vi "滑移力复检.vi"() -> ()   [LabVIEW 2020]
uses:
  <vilib>/Utility/miscctls.llb/LVRowAndColumnTypeDef.ctl
  Global_Variable/Global.vi
  Database/Global1.vi
  <vilib>/addons/database/Connection.llb/DB Tools Open Connec (String).vi
  Global_Variable/A131258.vi
  <vilib>/addons/database/Connection.llb/Conn Execute.vi
  <vilib>/addons/database/Recordset.llb/Rec Fetch Recordset Data (R).vi
  <vilib>/Utility/config.llb/NI_LVConfig.lvlib
  <vilib>/addons/database/NI_Database_API.lvlib
panel:
  out "判定":string[][](table)
  in  "滑移力判定项 2":string[][](table)
  out "连接的字符串 2":string
  out "连接的字符串":string
  out "时间":string
  out "前序工位":string[](array[string])
  out "二维码":string[][](array[string])
  out "传感器码":string[][](array[string])
  out "数组":refnum<vi>[](array[refnum])
  out "Fproductid_MAIN":string
  out "Fproductid_SENSOR":string
  out "USER_ID":string
  out "deviceid":string
  out "productid":string
  out "产品型号":string
  out "CODE_ID 2":string
  out "CODE_ID":string
  out "联机模式":string
  out "用户权限":string
  out "用户名":string
  in  "管柱合成报表":string[][](table)=[["mm"], ["mm/s"]]
  in  "拉轴判定结果":bool[][](array[boolean])=[[TRUE]]
  in  "滑移力判定结果":bool[][](array[boolean])=[[TRUE]]
  in  "管柱合成报表":string[][](table)=[["mm"], ["mm/s"]]
  in  "选项卡控件 2":enum32{"管柱总成装配", "管柱总成装配右", "滑移力曲线", "参数查看"}(tab)
  out "上柱管上序状态":string
  out "传感器上序状态":string
  out "上柱管上序状态":bool
  out "传感器上序状态":bool
  in  "质量报警":bool
  in  "设备缺料":bool
  in  "设备故障":bool
  out "产品条码":string
  out "不合格指示灯":bool
  out "合格指示灯":bool
  out "产品条码 3":string
  out "上柱管上序状态 3":string
  out "传感器上序状态 3":string
  out "上柱管上序状态 2":bool
  out "传感器上序状态 2":bool
  in  "质量报警2":bool
  in  "设备缺料2":bool
  in  "设备故障2":bool
  out "产品条码 2":string
  out "不合格指示灯":bool
  out "合格指示灯":bool
  out "产品条码 4":string
  out "装配结果":string
  out "管柱码状态":string
  out "传感器码状态":string
  out "管柱二维码":string
  out "传感器码":string
  out "滑移力复检曲线":cluster{dbl[], dbl[]}[](graph)
  out "表格控件":string[][](table)
  in  "删除":bool
  in  "确定":bool
  in  "添加":bool
  in  "退出":bool
  in  "更新":bool
  in  "产品型号":string(combo)
  in  "选项卡控件 3":enum32{"产品管理", "用户管理", "判定参数"}(tab)
  in  "请输入添加的产品名称":string
  in  "请选择要删除的产品":string(combo)
  in  "进入用户管理":bool
  in  "坐标参数":string[][](table)
  in  "滑移力判定项":string[][](table)
  in  "压力判定项":string[][](table)
  in  "判定项":string[][](table)=[["MM", "130", "180", ""], ["N", "-60", "-10", ""], ["N", "-60", "-10", ""], ["", "", "", ""], ["", "", "", ""], ["", "", "", ""]]
  # "滑移力复测及管柱总成装配台"
  # "产品二维码"
  # "生产结果"
  # "看板呼叫"
  # "壳体二维码"
  # "上序状态："
  # "上柱管二维码"
  # "上序状态："
  # "产品二维码"
  # "生产结果"
  # "看板呼叫"
  # "壳体二维码"
  # "上序状态："
  # "上柱管二维码"
  # "上序状态："
  # "装配结果"
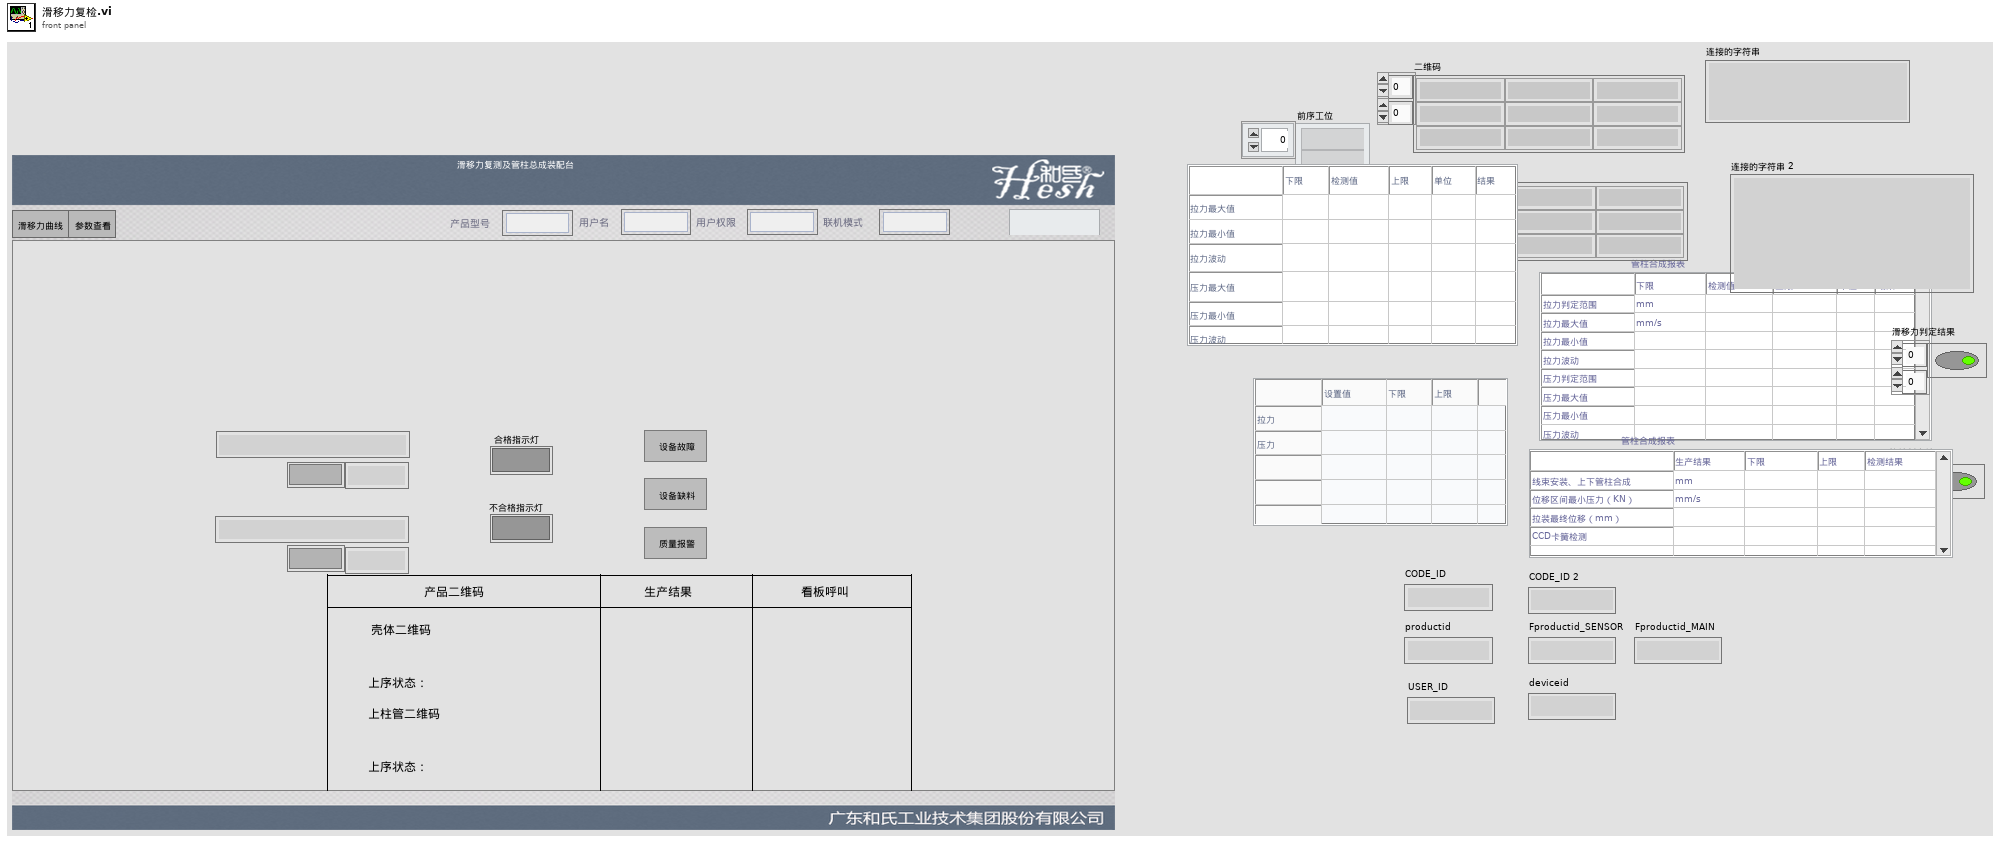
[diagram p1: front panel]
types:
  T1 = typedef "LVRowAndColumnTypeDef.ctl" = cluster{"Row":i32, "Column":i32}
  T2 = enum32{"Invalid", "Standard", "Closed", "Hidden", "Minimized", "Maximized"}
  T3 = cluster{"用户编号":string, "用户名":string, "用户密码(密文)":string, "用户权限":string}
  T4 = cluster{"设备名称":string, "用户名":string, "设备状态":enum16{"设备离线", "设备正常", "设备缺料", "设备故障", "质量报警"}, "附加信息":string}
  T5 = typedef "NI_LVConfig.lvlib/Config Data RefNum.ctl" = refnum<k1>
  T6 = typedef "NI_Database_API.lvlib/Conn ObjectReference.ctl" = refnum<k1>
  T7 = cluster{i64, i64, string, dbl, dbl, dbl, string, string}
  T8 = cluster{i64, i64, i64, string, "result string":string}
  T9 = cluster{i64, i64, i64, string, "result string":string}[]
  T10 = cluster{"拉力判定范围":cluster{"单位":string, "下限":dbl, "上限":dbl}, "拉力最大值":cluster{"单位":string, "下限":dbl, "上限":dbl}, "拉力最小值":cluster{"单位":string, "下限":dbl, "上限":dbl}, "拉力波动":cluster{"单位":string, "下限":dbl, "上限":dbl}, "压力判定范围":cluster{"单位":string, "下限":dbl, "上限":dbl}, "压力最大值":cluster{"单位":string, "下限":dbl, "上限":dbl}, "压力最小值":cluster{"单位":string, "下限":dbl, "上限":dbl}, "压力波动":cluster{"单位":string, "下限":dbl, "上限":dbl}}
  T11 = cluster{i64, i64, string, dbl, dbl, dbl, string, string}[]
  T12 = typedef "NI_Database_API.lvlib/Rec ObjectReference.ctl" = refnum<k1>
  T13 = cluster{"[0]":cluster{string, dbl, dbl}, "[1]":cluster{string, dbl, dbl}, "[2]":cluster{string, dbl, dbl}, "[3]":cluster{string, dbl, dbl}, "[4]":cluster{string, dbl, dbl}, "[5]":cluster{string, dbl, dbl}, "[6]":cluster{string, dbl, dbl}, "[7]":cluster{string, dbl, dbl}}
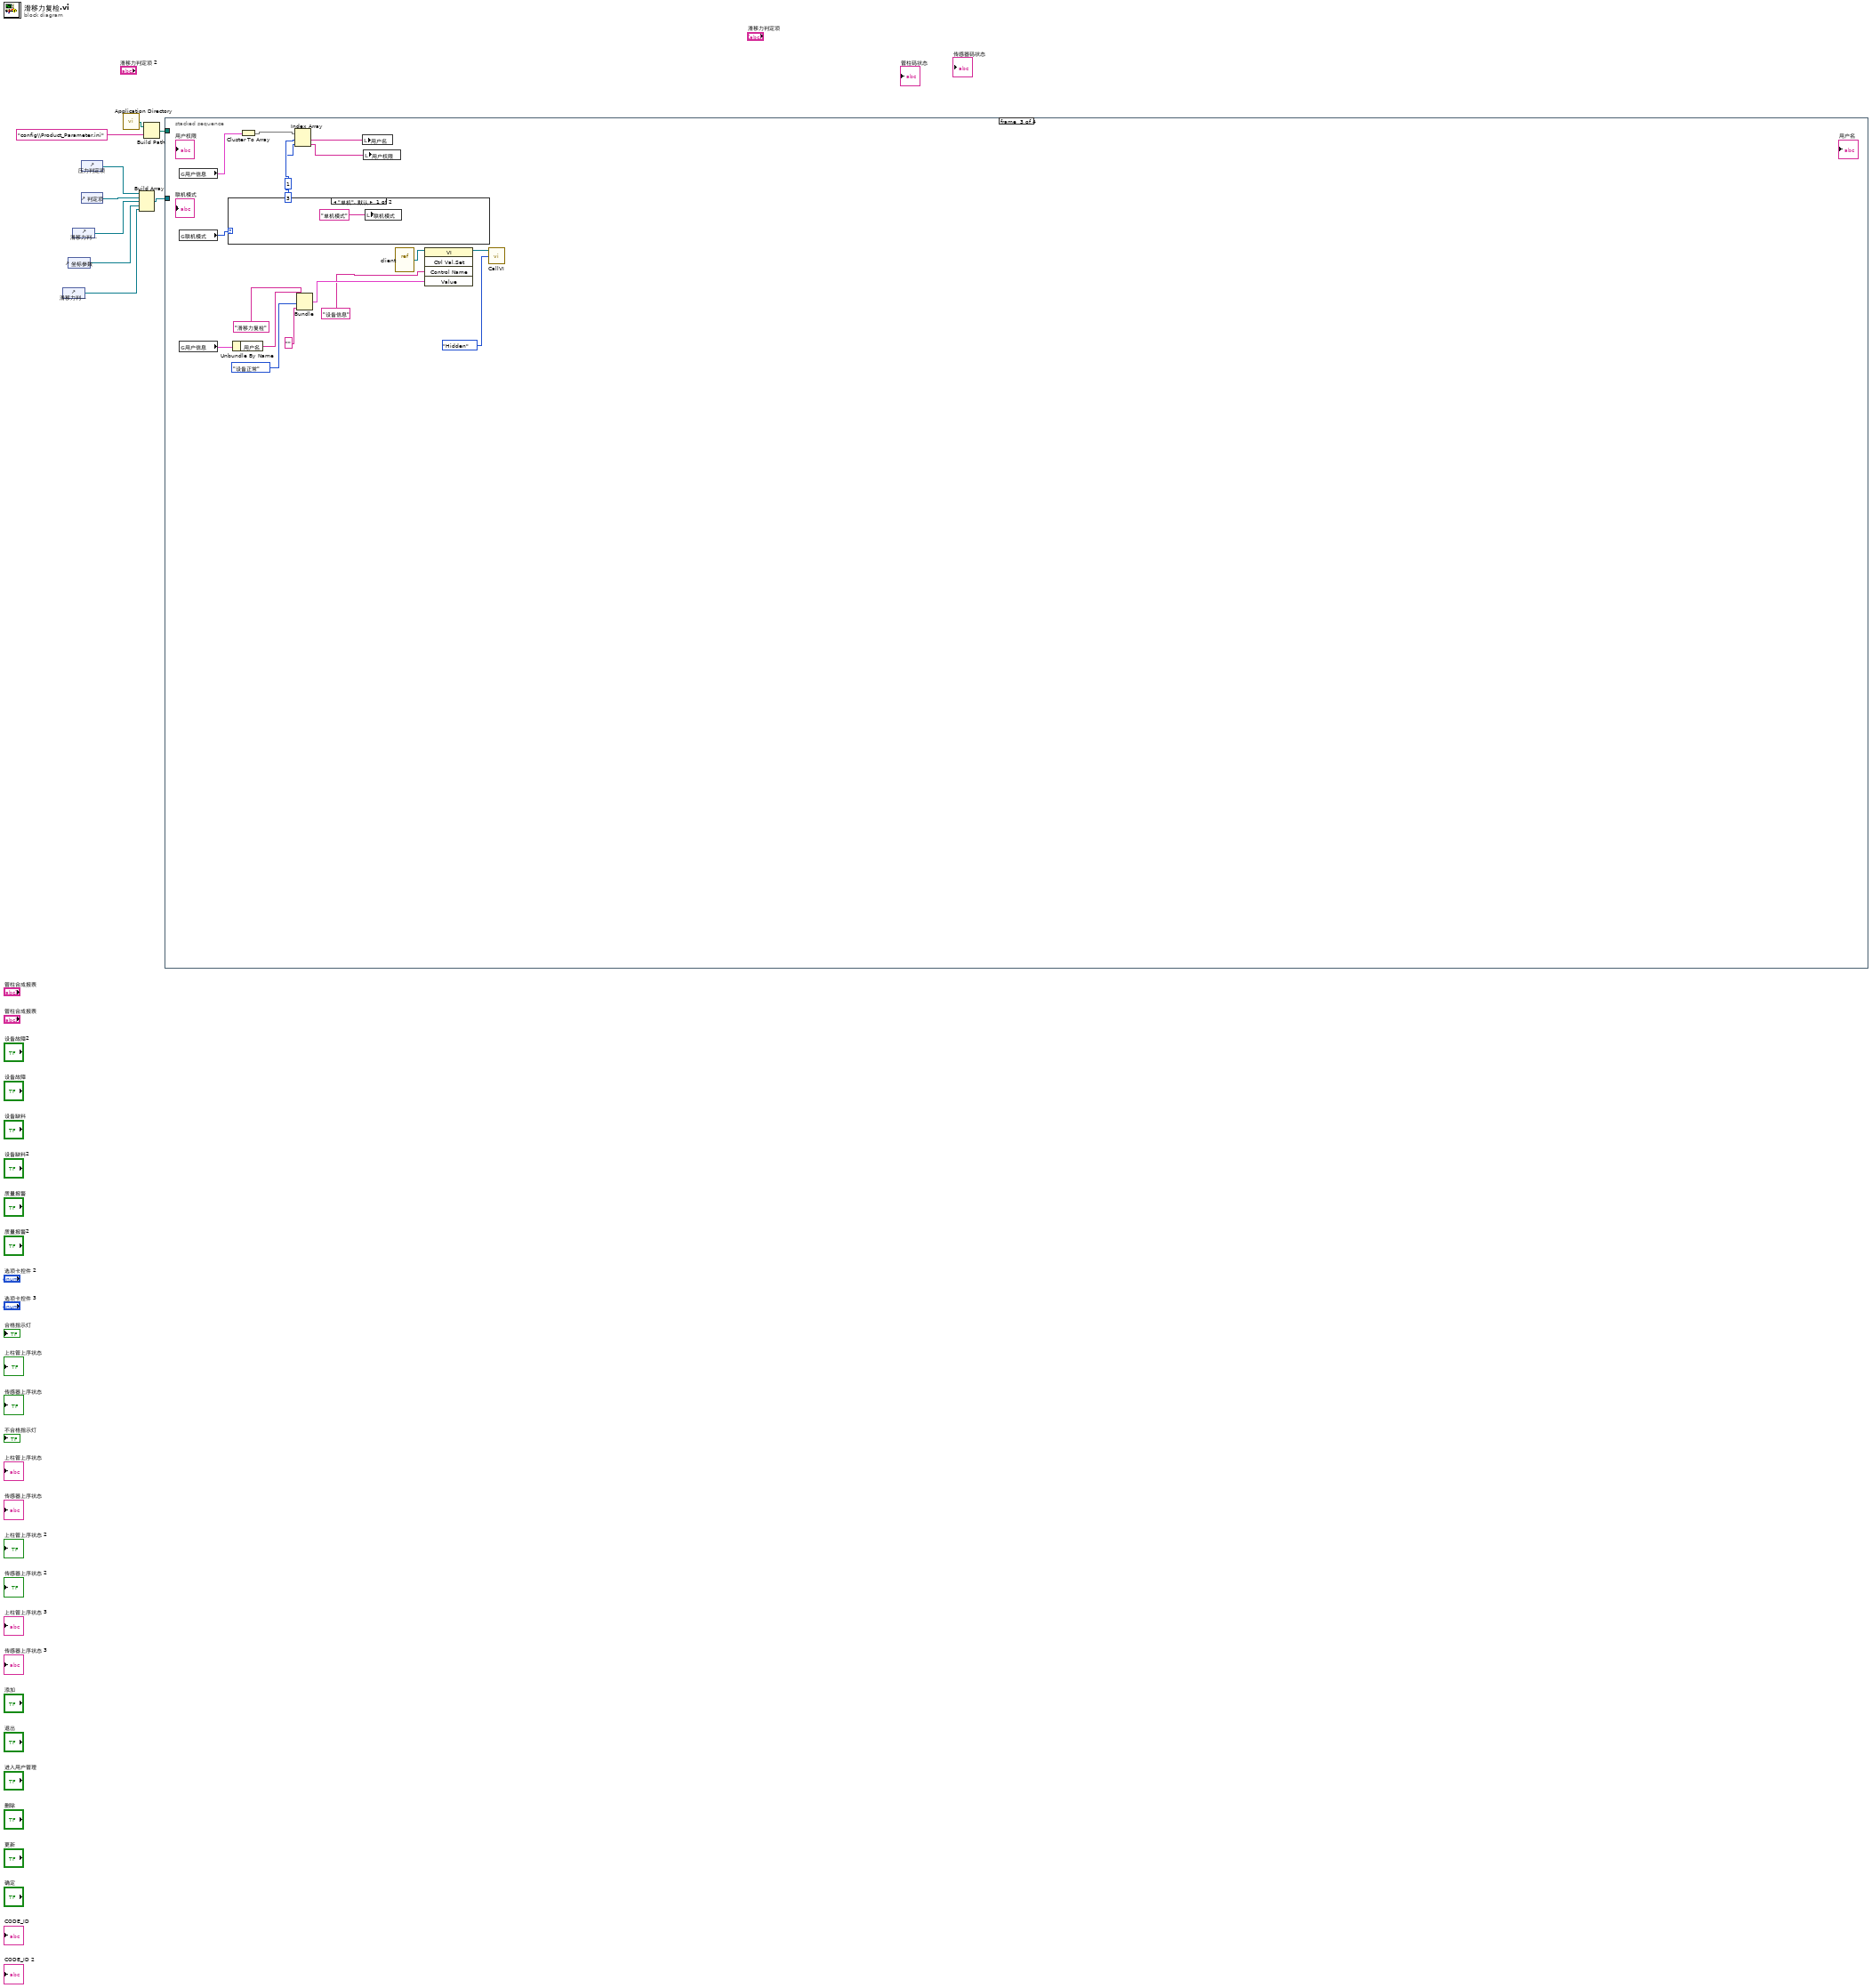
[diagram p0: block diagram]
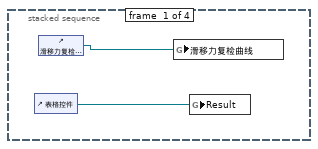
[diagram p2: hidden frame]
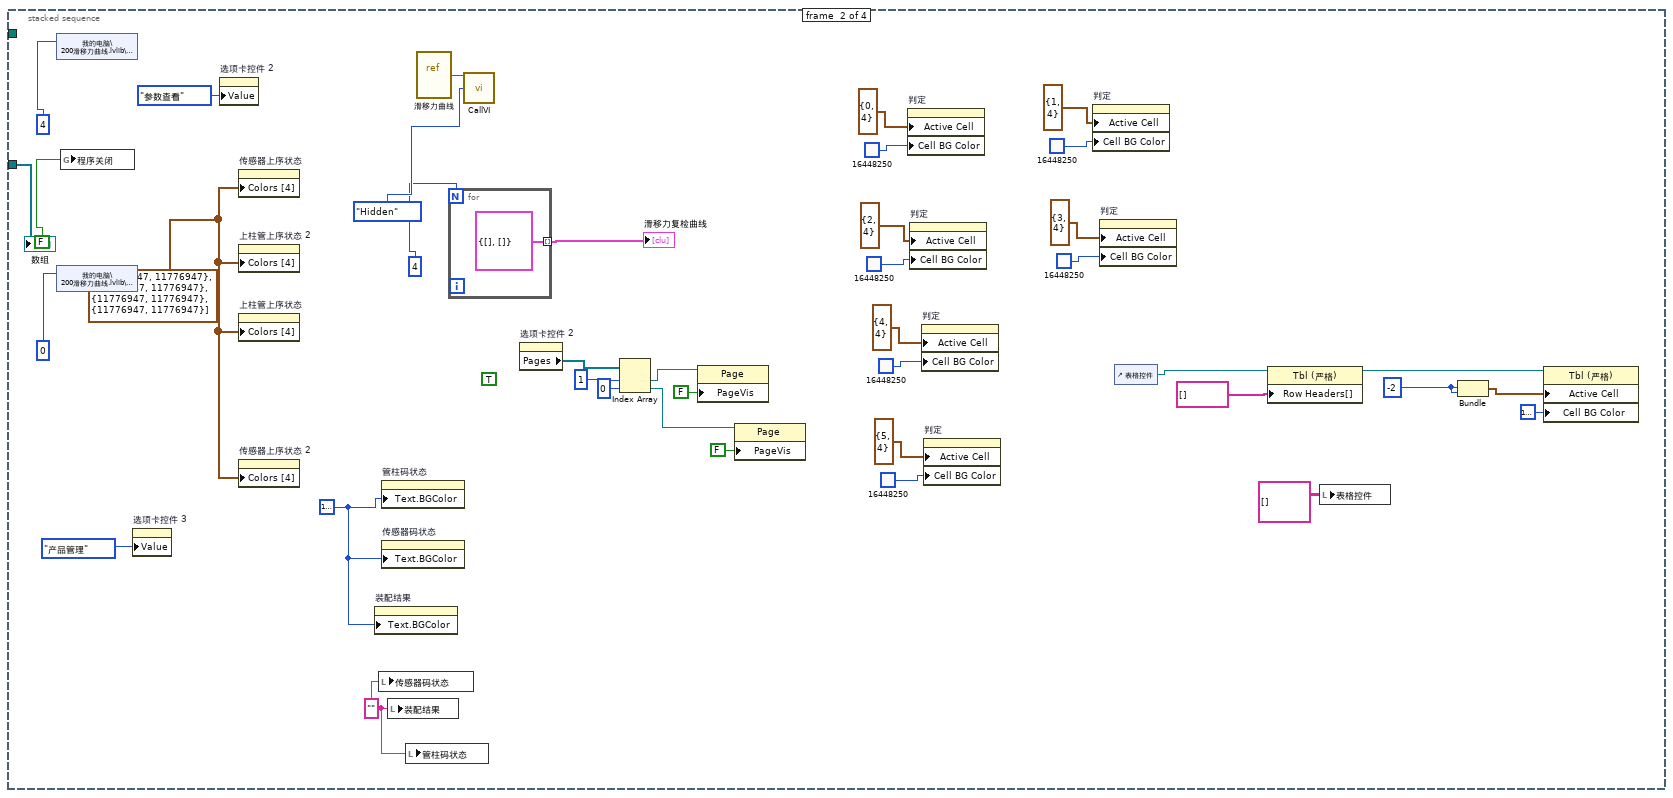
[diagram p3: hidden frame]
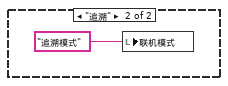
[diagram p4: hidden frame]
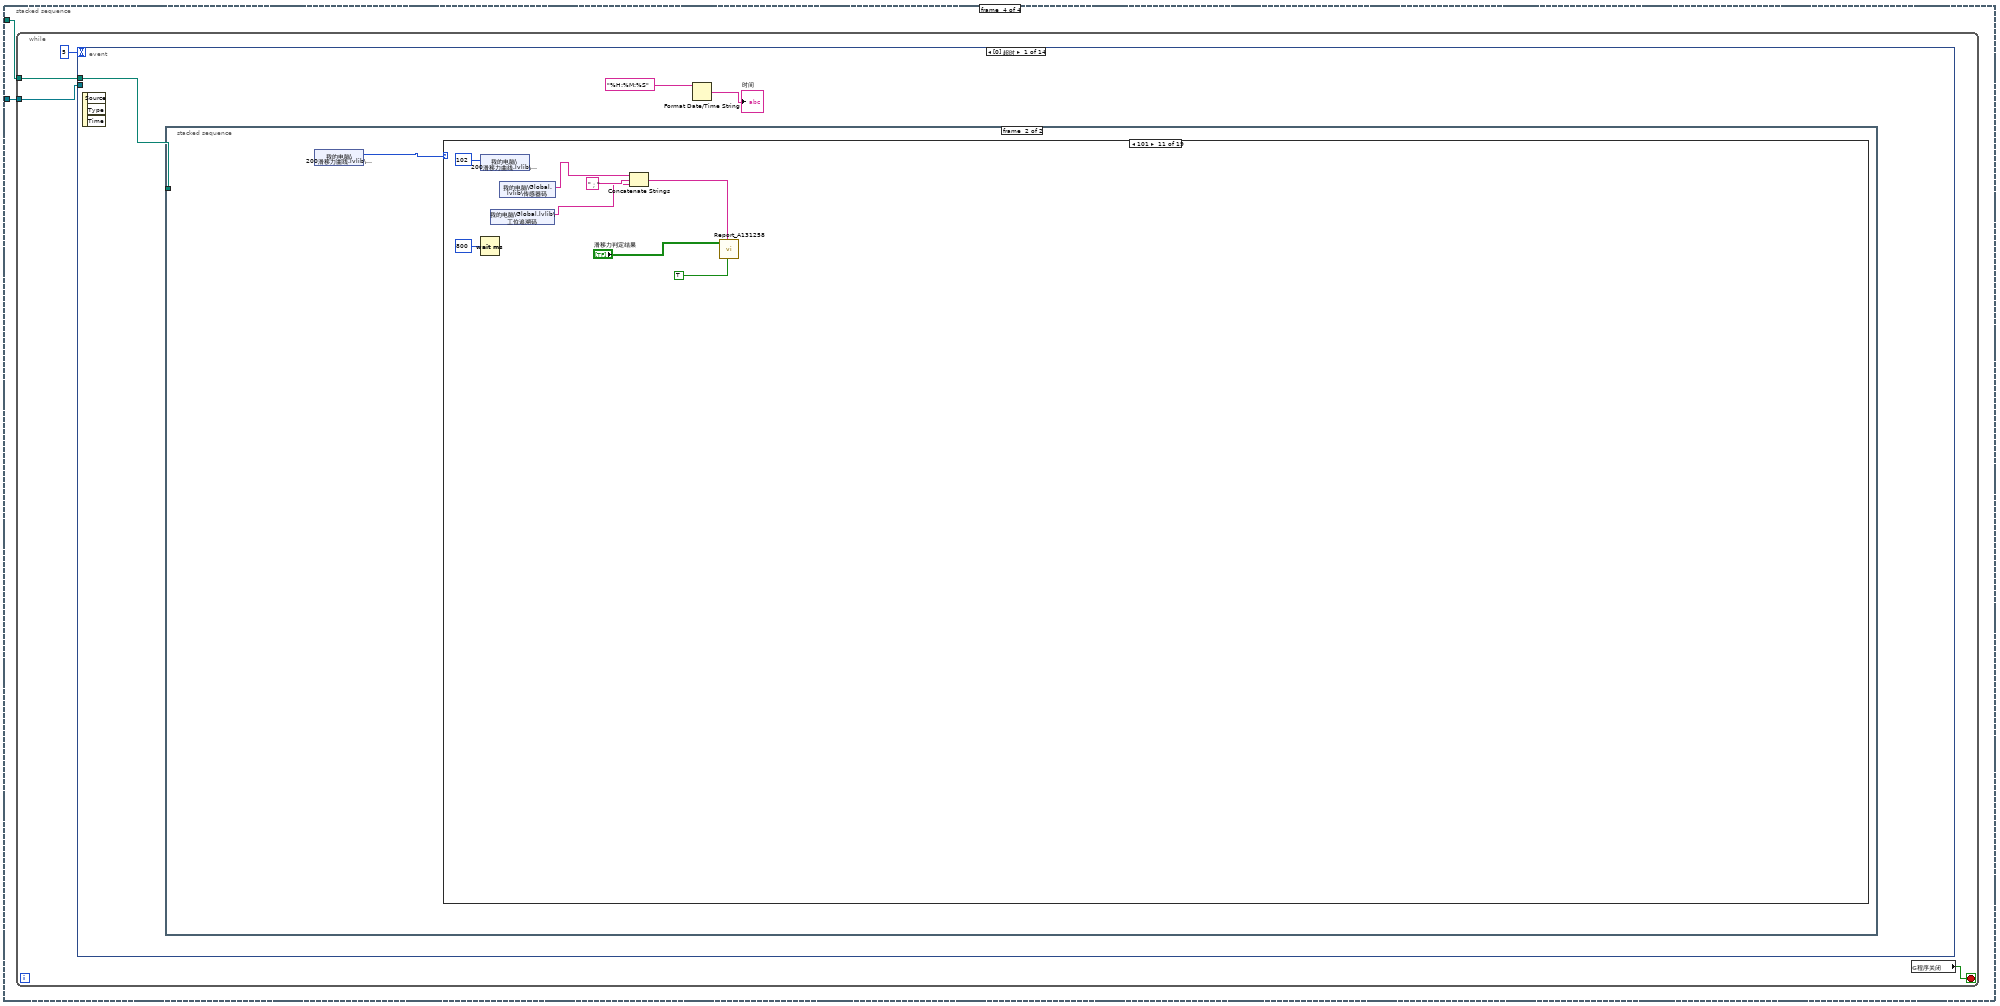
[diagram p5: hidden frame]
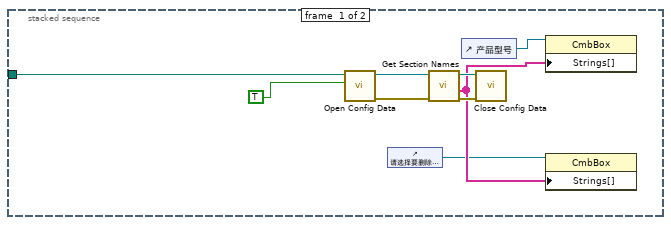
[diagram p6: hidden frame]
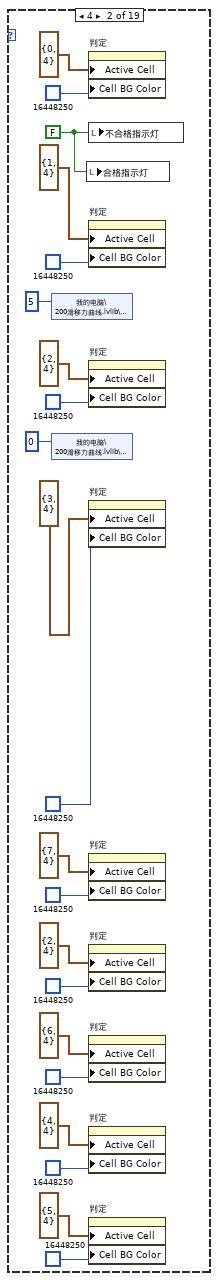
[diagram p8: hidden frame]
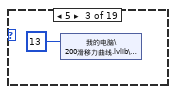
[diagram p9: hidden frame]
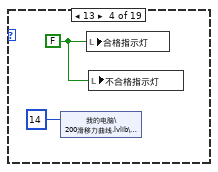
[diagram p10: hidden frame]
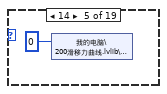
[diagram p11: hidden frame]
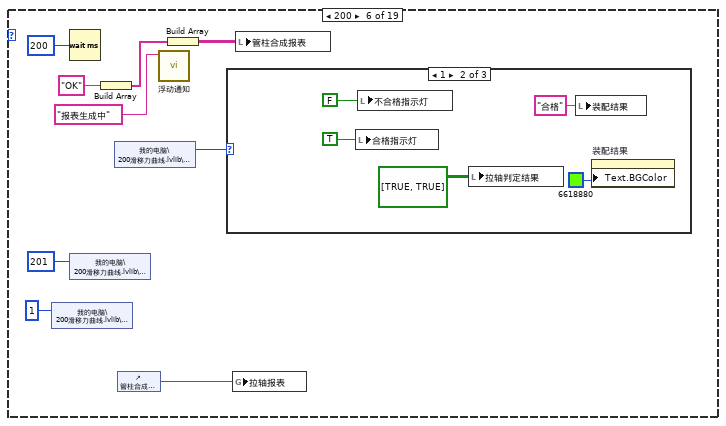
[diagram p12: hidden frame]
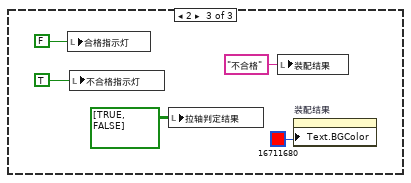
[diagram p14: hidden frame]
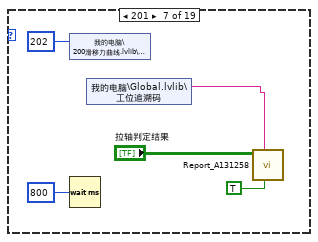
[diagram p15: hidden frame]
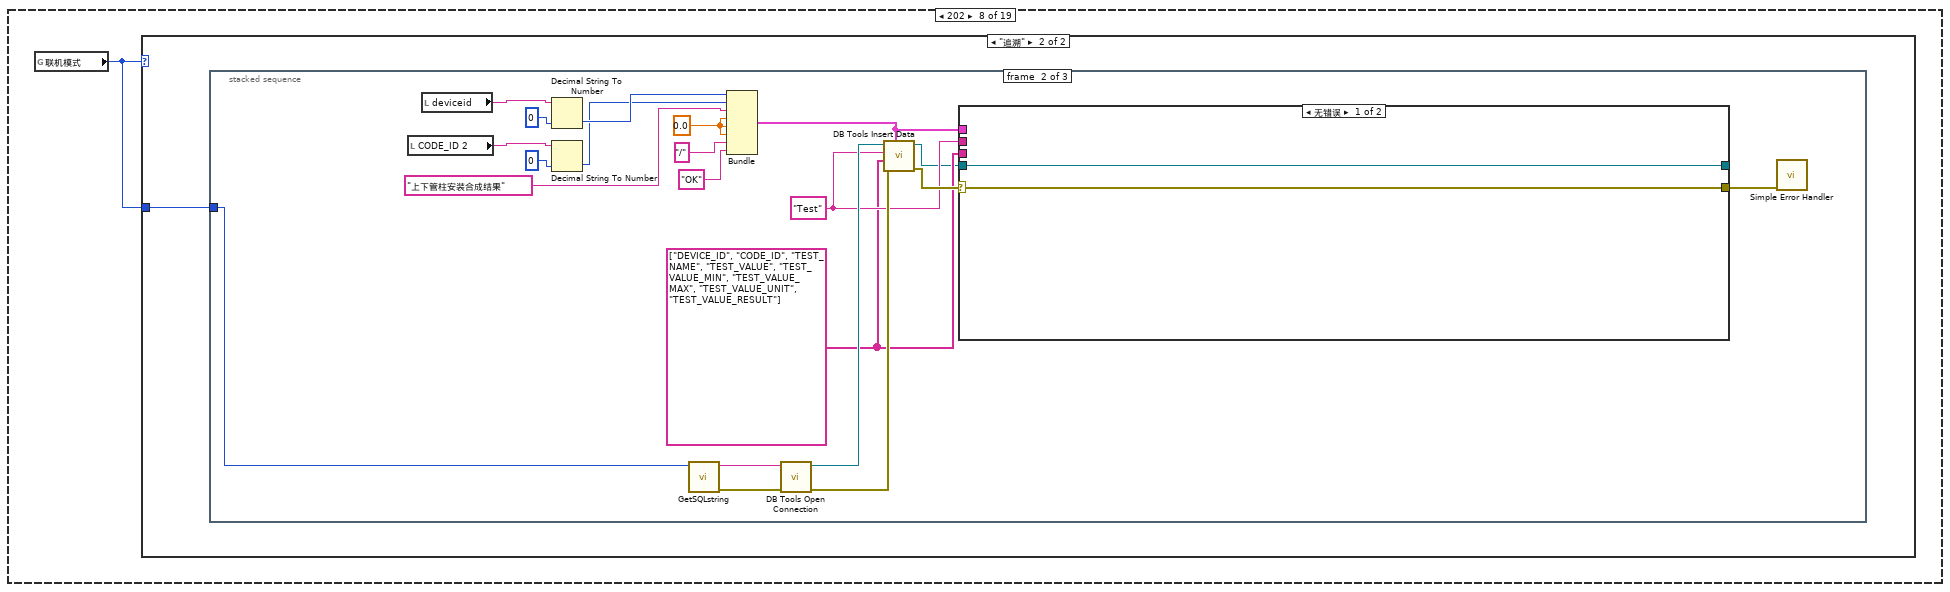
[diagram p16: hidden frame]
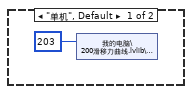
[diagram p17: hidden frame]
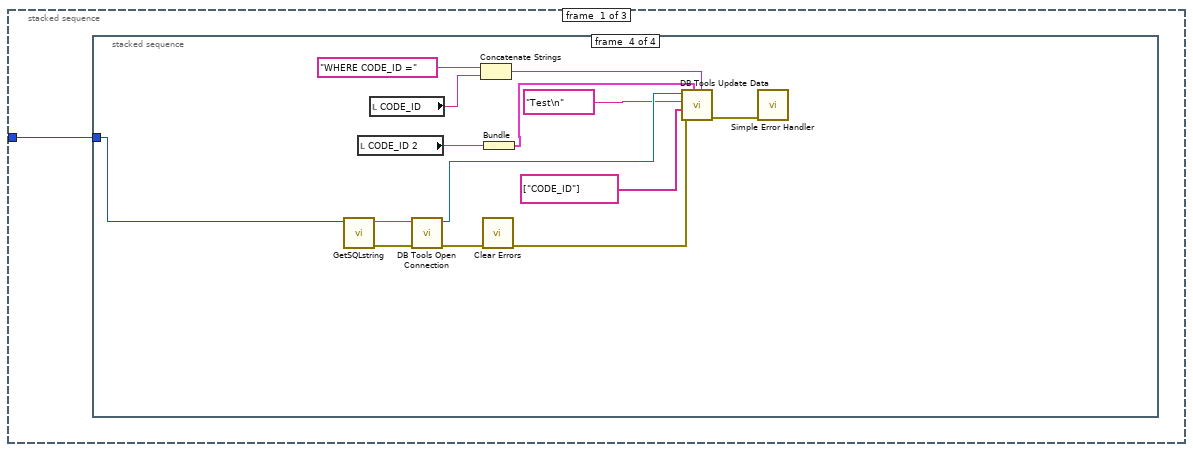
[diagram p18: hidden frame]
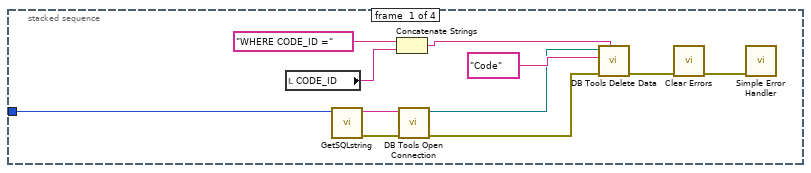
[diagram p19: hidden frame]
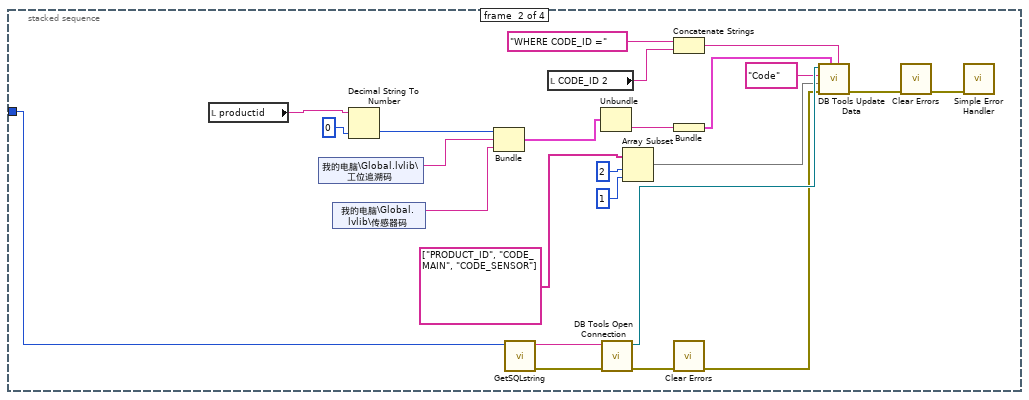
[diagram p20: hidden frame]
diagram:
  n1 = control-ref of="滑移力判定项 2"() -> (w1:refnum<vi>)
  n2 = control-ref of="坐标参数"() -> (w2:refnum<vi>)
  n3 = control-ref of="滑移力判定项"() -> (w3:refnum<vi>)
  n4 = control-ref of="压力判定项"() -> (w5:refnum<vi>)
  n5 = control-ref of="判定项"() -> (w4:refnum<vi>)
  n6 = call <vilib>:"Application Directory.vi"() -> ("Application Directory"=w7:path)
  n7 = Build Array(w5, w4, w3, w2, w1) -> (w6:refnum<vi>[])
  n8 = Build Path(base path=w7, name or relative path="config\\Product_Parameter.ini" ("名称或相对路径")) -> (appended path=w8:path)
  n9 = stacked-sequence {
    tunnel: w8 -> [_ _ _ w72]
    tunnel: w6 -> [_ w45 _ w71]
    frame #0 {
      n10 = control-ref of="表格控件"() -> (w10:refnum<vi>)
      n11 = control-ref of="滑移力复检曲线"() -> (w11:refnum<vi>)
      n12 = global write "Global.vi" "滑移力复检曲线"(w11) -> ()
      n13 = global write "Global.vi" "Result"(w10) -> ()
    }
    frame #1 {
      w13 = -2
      w31 = "" ("装配结果")
      (unwired) TRUE ("页选择器可见")
      w32 = u32 16777216
      w47 = cluster{u32, u32}[] [{11776947, 11776947}, {11776947, 11776947}, {11776947, 11776947}, {11776947, 11776947}] ("颜色[4]")
      n14 = shared-variable "我的电脑\\200滑移力曲线.lvlib\\备用_1"(4) -> ()  [unwired: 1 in, 1 out]
      n15 = shared-variable "我的电脑\\200滑移力曲线.lvlib\\备用_3"(u16 0 ("备用1")) -> ()  [unwired: 1 in, 1 out]
      n16 = global write "Global.vi" "程序关闭"(FALSE ("程序关闭")) -> ()
      n17 = property on="选项卡控件 3" class="TabCtl (严格)"("Value"=enum32{"产品管理", "用户管理"}."产品管理" ("选项卡控件 3")) -> ()  [unwired: 2 in, 2 out]
      n18 = property on="选项卡控件 2" class="TabCtl (严格)"("Value"=enum32{"管柱总成装配", "管柱总成装配右", "滑移力曲线", "参数查看"}."参数查看" ("选项卡控件 2")) -> ()  [unwired: 2 in, 2 out]
      n19 = property on="传感器上序状态" class="Bool (严格)"("Colors [4]"=w47) -> ()  [unwired: 2 in, 2 out]
      n20 = property on="上柱管上序状态 2" class="Bool (严格)"("Colors [4]"=w47) -> ()  [unwired: 2 in, 2 out]
      n21 = property on="上柱管上序状态" class="Bool (严格)"("Colors [4]"=w47) -> ()  [unwired: 2 in, 2 out]
      n22 = property on="传感器上序状态 2" class="Bool (严格)"("Colors [4]"=w47) -> ()  [unwired: 2 in, 2 out]
      n23 = property on="装配结果" class="Str"("Text.BGColor"=w32) -> ()  [unwired: 2 in, 2 out]
      n24 = local write "传感器码状态"(w31) -> ()
      n25 = property on="管柱码状态" class="Str"("Text.BGColor"=w32) -> ()  [unwired: 2 in, 2 out]
      n26 = property on="传感器码状态" class="Str"("Text.BGColor"=w32) -> ()  [unwired: 2 in, 2 out]
      n27 = local write "装配结果"(w31) -> ()
      n28 = local write "管柱码状态"(w31) -> ()
      n29 = vi-ref "滑移力曲线.vi"() -> (w44:refnum<vi>)
      n30 = for {
        N: 4 -> [_]
        tunnel: [cluster{dbl[], dbl[]} {[], []}] -> w42 mode=indexing
      }
      "滑移力复检曲线" <- w42
      n31 = call "CallVI.vi"("VI引用"=w44, "状态"=T2."Hidden") -> ()  [unwired: 12 in, 2 out]
      n32 = property on="选项卡控件 2" class="TabCtl (严格)"() -> ("Pages"=w39:refnum<vi>[])  [unwired: 2 in, 2 out]
      n33 = Index Array(array=w39, index #1=1 ("索引"), index #2=0 ("索引")) -> (element #1=w38:refnum<vi>, element #2=w34:refnum<vi>)
      n34 = property class="Page"(reference=w38, "PageVis"=FALSE ("选项卡可见")) -> ()  [unwired: 1 in, 2 out]
      n35 = property class="Page"(reference=w34, "PageVis"=FALSE ("选项卡可见")) -> ()  [unwired: 1 in, 2 out]
      n36 = property on="判定" class="Tbl (严格)"("Active Cell"=T1 {"Row"=0, "Column"=4} ("活动单元格:活动单元格"), "Cell BG Color"=u32 16448250) -> ()  [unwired: 2 in, 2 out]
      n37 = property on="判定" class="Tbl (严格)"("Active Cell"=T1 {"Row"=2, "Column"=4} ("活动单元格:活动单元格"), "Cell BG Color"=u32 16448250) -> ()  [unwired: 2 in, 2 out]
      n38 = property on="判定" class="Tbl (严格)"("Active Cell"=T1 {"Row"=4, "Column"=4} ("活动单元格:活动单元格"), "Cell BG Color"=u32 16448250) -> ()  [unwired: 2 in, 2 out]
      n39 = property on="判定" class="Tbl (严格)"("Active Cell"=T1 {"Row"=5, "Column"=4} ("活动单元格:活动单元格"), "Cell BG Color"=u32 16448250) -> ()  [unwired: 2 in, 2 out]
      n40 = property on="判定" class="Tbl (严格)"("Active Cell"=T1 {"Row"=1, "Column"=4} ("活动单元格:活动单元格"), "Cell BG Color"=u32 16448250) -> ()  [unwired: 2 in, 2 out]
      n41 = property on="判定" class="Tbl (严格)"("Active Cell"=T1 {"Row"=3, "Column"=4} ("活动单元格:活动单元格"), "Cell BG Color"=u32 16448250) -> ()  [unwired: 2 in, 2 out]
      n42 = control-ref of="表格控件"() -> (w18:refnum<vi>)
      n43 = property class="Tbl (严格)"(reference=w18, "Row Headers[]"=string[] [] ("行首字符串[]")) -> (reference out=w16:refnum<vi>)  [unwired: 1 in, 1 out]
      n44 = local write "表格控件"(string[][] [] ("表格控件")) -> ()
      n45 = Bundle(w13, w13) -> (w14:cluster{i32, i32})  [unwired: 1 in]
      n46 = property class="Tbl (严格)"(reference=w16, "Active Cell"=w14, "Cell BG Color"=u32 16777216 ("活动单元格:单元格背景色")) -> ()  [unwired: 1 in, 2 out]
      "数组" <- w45
    }
    frame #2 {
      n47 = global read "Global1.vi" "用户信息"() -> (w68:T3)
      n48 = global read "Global1.vi" "联机模式"() -> (w62:enum16{"单机", "追溯"})
      n49 = global read "Global1.vi" "用户信息"() -> (w59:T3)
      n50 = case shown="\"单机\", 默认" w62 {
        frame "单机", Default {
          n51 = local write "联机模式"("单机模式" ("联机模式")) -> ()
        }
        frame "追溯" {
          n52 = local write "联机模式"("追溯模式" ("联机模式")) -> ()
        }
      }
      n53 = Unbundle By Name(w59) -> ("用户名"=w58:string)
      n54 = Cluster To Array(cluster=w68) -> (array=w67:string[])
      n55 = Index Array(array=w67, index #1=1 ("索引"), index #2=3 ("索引")) -> (element #1=w64:string, element #2=w63:string)
      n56 = Bundle("设备名称"="滑移力复检", "用户名"=w58, "设备状态"=enum16{"设备离线", "设备正常", "设备缺料", "设备故障", "质量报警"}."设备正常", "附加信息"="") -> (w57:T4)  [unwired: 1 in]
      n57 = local write "用户名"(w64) -> ()
      n58 = local write "用户权限"(w63) -> ()
      n59 = vi-ref "client.vi"() -> (w61:refnum<vi>)
      n60 = invoke class="VI" method="Ctrl Val.Set"(reference=w61, "Control Name"="设备信息" ("控件名"), "Value"=w57) -> (reference out=w60:refnum<vi>)  [unwired: 2 in, 4 out]
      n61 = call "CallVI.vi"("VI引用"=w60, "状态"=T2."Hidden") -> ()  [unwired: 12 in, 2 out]
    }
    frame #3 {
      n62 = while {
        tunnel: w72 -> [w75]
        tunnel: w71 -> [w73]
        stop <- w74 stop-if-true
        n63 = event shown="[0] 超时" {
          selector: _ -> [_ _ _ _ _ _ _ _ _ _ _ _ _ _]
          dyn-events: _ -> [_ _ _ _ _ _ _ _ _ _ _ _ _ _]
          timeout: 5 -> [_ _ _ _ _ _ _ _ _ _ _ _ _ _]
          tunnel: w75 -> [w79 w859 _ w1025 w1044 _ w1055 _ _ _ _ _ _ w1097]
          tunnel: w73 -> [_ _ _ w1023 w1043 _ w1054 _ _ _ _ _ _ _]
          event Timeout {
            n64 = event-data() -> ()  [unwired: 1 in, 3 out]
            n65 = stacked-sequence {
              tunnel: w79 -> [w88 _]
              frame #0 {
                n66 = call <vilib>:"Open Config Data.vi"("create file if necessary (T)"=TRUE, "configuration file path"=w88) -> ("error out"=w85:errorcluster, "refnum"=w84:T5)  [unwired: 7 in, 1 out]
                n67 = control-ref of="请选择要删除的产品"() -> (w81:refnum<vi>)
                n68 = call <vilib>:"Get Section Names.vi"("error in (no error)"=w85, "refnum"=w84) -> ("error out"=w87:errorcluster, "section names"=w83:string[], "refnum out"=w86:T5)  [unwired: 7 in]
                n69 = control-ref of="产品型号"() -> (w82:refnum<vi>)
                n70 = call <vilib>:"Close Config Data.vi"("error in (no error)"=w87, "refnum"=w86) -> ()  [unwired: 8 in, 2 out]
                n71 = property on="属性节点" class="CmbBox"(reference=w82, "Strings[]"=w83) -> ()  [unwired: 1 in, 2 out]
                n72 = property on="属性节点" class="CmbBox"(reference=w81, "Strings[]"=w83) -> ()  [unwired: 1 in, 2 out]
              }
              frame #1 {
                n73 = shared-variable "我的电脑\\200滑移力曲线.lvlib\\备用_1"() -> (w89:u16)  [unwired: 1 in, 1 out]
                n74 = case shown="101" w89 {
                  frame 0, Default {
                  }
                  frame 4 {
                    w109 = FALSE
                    n75 = shared-variable "我的电脑\\200滑移力曲线.lvlib\\备用_1"(5) -> ()  [unwired: 1 in, 1 out]
                    n76 = shared-variable "我的电脑\\200滑移力曲线.lvlib\\备用_3"(u16 0 ("备用1")) -> ()  [unwired: 1 in, 1 out]
                    n77 = local write "合格指示灯"(w109) -> ()
                    n78 = property on="判定" class="Tbl (严格)"("Active Cell"=T1 {"Row"=0, "Column"=4} ("活动单元格:活动单元格"), "Cell BG Color"=u32 16448250) -> ()  [unwired: 2 in, 2 out]
                    n79 = local write "不合格指示灯"(w109) -> ()
                    n80 = property on="判定" class="Tbl (严格)"("Active Cell"=T1 {"Row"=1, "Column"=4} ("活动单元格:活动单元格"), "Cell BG Color"=u32 16448250) -> ()  [unwired: 2 in, 2 out]
                    n81 = property on="判定" class="Tbl (严格)"("Active Cell"=T1 {"Row"=2, "Column"=4} ("活动单元格:活动单元格"), "Cell BG Color"=u32 16448250) -> ()  [unwired: 2 in, 2 out]
                    n82 = property on="判定" class="Tbl (严格)"("Active Cell"=T1 {"Row"=3, "Column"=4} ("活动单元格:活动单元格"), "Cell BG Color"=u32 16448250) -> ()  [unwired: 2 in, 2 out]
                    n83 = property on="判定" class="Tbl (严格)"("Active Cell"=T1 {"Row"=7, "Column"=4} ("活动单元格:活动单元格"), "Cell BG Color"=u32 16448250) -> ()  [unwired: 2 in, 2 out]
                    n84 = property on="判定" class="Tbl (严格)"("Active Cell"=T1 {"Row"=2, "Column"=4} ("活动单元格:活动单元格"), "Cell BG Color"=u32 16448250) -> ()  [unwired: 2 in, 2 out]
                    n85 = property on="判定" class="Tbl (严格)"("Active Cell"=T1 {"Row"=6, "Column"=4} ("活动单元格:活动单元格"), "Cell BG Color"=u32 16448250) -> ()  [unwired: 2 in, 2 out]
                    n86 = property on="判定" class="Tbl (严格)"("Active Cell"=T1 {"Row"=4, "Column"=4} ("活动单元格:活动单元格"), "Cell BG Color"=u32 16448250) -> ()  [unwired: 2 in, 2 out]
                    n87 = property on="判定" class="Tbl (严格)"("Active Cell"=T1 {"Row"=5, "Column"=4} ("活动单元格:活动单元格"), "Cell BG Color"=u32 16448250) -> ()  [unwired: 2 in, 2 out]
                  }
                  frame 5 {
                    n88 = shared-variable "我的电脑\\200滑移力曲线.lvlib\\备用_1"(13) -> ()  [unwired: 1 in, 1 out]
                  }
                  frame 13 {
                    w112 = FALSE
                    n89 = shared-variable "我的电脑\\200滑移力曲线.lvlib\\备用_1"(14) -> ()  [unwired: 1 in, 1 out]
                    n90 = local write "合格指示灯"(w112) -> ()
                    n91 = local write "不合格指示灯"(w112) -> ()
                  }
                  frame 14 {
                    n92 = shared-variable "我的电脑\\200滑移力曲线.lvlib\\备用_1"(0) -> ()  [unwired: 1 in, 1 out]
                  }
                  frame 200 {
                    n93 = shared-variable "我的电脑\\200滑移力曲线.lvlib\\备用_3"(u16 1 ("备用1")) -> ()  [unwired: 1 in, 1 out]
                    n94 = Wait (ms)(milliseconds to wait=u32 200 ("等待时间（毫秒）")) -> ()  [unwired: 1 out]
                    n95 = shared-variable "我的电脑\\200滑移力曲线.lvlib\\备用_1"(u16 201 ("备用1")) -> ()  [unwired: 1 in, 1 out]
                    n96 = Build Array("OK") -> (w115:string[])
                    n97 = shared-variable "我的电脑\\200滑移力曲线.lvlib\\备用_8"() -> (w119:u16)  [unwired: 1 in, 1 out]
                    n98 = control-ref of="管柱合成报表"() -> (w120:refnum<vi>)
                    n99 = call "浮动通知.vi"("通知内容"="报表生成中" ("Status")) -> ()  [unwired: 11 in]
                    n100 = Build Array(w115) -> (w122:string[][])
                    n101 = case shown="1" w119 {
                      frame 0, Default {
                      }
                      frame 1 {
                        n102 = local write "合格指示灯"(TRUE) -> ()
                        n103 = local write "不合格指示灯"(FALSE ("不合格指示灯")) -> ()
                        n104 = local write "拉轴判定结果"(bool[][] [[TRUE, TRUE]] ("判定结果")) -> ()
                        n105 = local write "装配结果"("合格" ("装配结果")) -> ()
                        n106 = property on="装配结果" class="Str"("Text.BGColor"=u32 6618880 ("文本.文本颜色:背景色")) -> ()  [unwired: 2 in, 2 out]
                      }
                      frame 2 {
                        n107 = local write "合格指示灯"(FALSE ("合格指示灯")) -> ()
                        n108 = local write "不合格指示灯"(TRUE) -> ()
                        n109 = local write "拉轴判定结果"(bool[][] [[TRUE, FALSE]] ("判定结果")) -> ()
                        n110 = local write "装配结果"("不合格" ("装配结果")) -> ()
                        n111 = property on="装配结果" class="Str"("Text.BGColor"=u32 16711680 ("文本.文本颜色:背景色")) -> ()  [unwired: 2 in, 2 out]
                      }
                    }
                    n112 = global write "Global.vi" "拉轴报表"(w120) -> ()
                    n113 = local write "管柱合成报表"(w122) -> ()
                  }
                  frame 201 {
                    n114 = shared-variable "我的电脑\\200滑移力曲线.lvlib\\备用_1"(u16 202 ("备用1")) -> ()  [unwired: 1 in, 1 out]
                    n115 = Wait (ms)(milliseconds to wait=u32 800 ("等待时间（毫秒）")) -> ()  [unwired: 1 out]
                    n116 = shared-variable "我的电脑\\Global.lvlib\\工位追溯码"() -> (w134:string)  [unwired: 1 in, 1 out]
                    n117 = call "Report_A131258.vi"("文件重命名"=TRUE, "文件名称"=w134, "布尔数组"="拉轴判定结果") -> ()  [unwired: 8 in, 1 out]
                  }
                  frame 202 {
                    n118 = global read "Global1.vi" "联机模式"() -> (w139:enum16{"单机", "追溯"})
                    n119 = case shown="\"追溯\"" w139 {
                      tunnel: w139 -> [_ w141]
                      frame "单机", Default {
                        n120 = shared-variable "我的电脑\\200滑移力曲线.lvlib\\备用_1"(u16 203 ("备用1")) -> ()  [unwired: 1 in, 1 out]
                      }
                      frame "追溯" {
                        n121 = stacked-sequence {
                          tunnel: w141 -> [w142 w212 _]
                          frame #0 {
                            n122 = stacked-sequence {
                              tunnel: w142 -> [w147 w156 w178 w192]
                              frame #0 {
                                n123 = local read "CODE_ID"() -> (w153:string)
                                n124 = call "GetSQLstring.vi"("联机模式"=w147) -> ("错误输出"=w149:errorcluster, "连接字符串"=w148:string)  [unwired: 9 in]
                                n125 = Concatenate Strings("WHERE CODE_ID =" ("condition"), w153) -> (w152:string)
                                n126 = call-poly <vilib>:"DB Tools Open Connection.vi"("error in (no error)"=w149, "connection information"=w148) -> ("error out"=w145:errorcluster, "connection reference"=w146:T6)  [unwired: 6 in]
                                n127 = call <vilib>:"DB Tools Delete Data.vi"("condition"=w152, "error in (no error)"=w145, "table"="Code", "connection reference"=w146) -> ("error out"=w144:errorcluster)  [unwired: 6 in, 1 out]
                                n128 = call <vilib>:"Clear Errors.vi"("error in (no error)"=w144) -> ("error out"=w143:errorcluster)  [unwired: 5 in, 1 out]
                                n129 = call <vilib>:"Simple Error Handler.vi"("error in (no error)"=w143) -> ()  [unwired: 4 in, 5 out]
                              }
                              frame #1 {
                                n130 = local read "productid"() -> (w168:string)
                                n131 = shared-variable "我的电脑\\Global.lvlib\\工位追溯码"() -> (w165:string)  [unwired: 1 in, 1 out]
                                n132 = shared-variable "我的电脑\\Global.lvlib\\传感器码"() -> (w166:string)  [unwired: 1 in, 1 out]
                                n133 = Decimal String To Number(string=w168, default (0L)=i64 0 ("默认(0 I32)")) -> (number=w169:i64)  [unwired: 1 in, 1 out]
                                n134 = Bundle(w169, "String"=w165, "String"=w166) -> (w167:cluster{i64, "String":string, "String":string})  [unwired: 1 in]
                                n135 = call "GetSQLstring.vi"("联机模式"=w156) -> ("错误输出"=w164:errorcluster, "连接字符串"=w163:string)  [unwired: 9 in]
                                n136 = local read "CODE_ID 2"() -> (w177:string)
                                n137 = Unbundle(w167) -> ("String"=w174:string)  [unwired: 2 out]
                                n138 = call-poly <vilib>:"DB Tools Open Connection.vi"("error in (no error)"=w164, "connection information"=w163) -> ("error out"=w176:errorcluster, "connection reference"=w175:T6)  [unwired: 6 in]
                                n139 = Array Subset(array=string[] ["PRODUCT_ID", "CODE_MAIN", "CODE_SENSOR"] ("columns"), index=2 ("长度"), length=1 ("索引")) -> (w171:string[])
                                n140 = Concatenate Strings("WHERE CODE_ID =" ("condition"), w177) -> (w172:string)
                                n141 = Bundle("String"=w174) -> (w173:cluster{"String":string})  [unwired: 1 in]
                                n142 = call <vilib>:"Clear Errors.vi"("error in (no error)"=w176) -> ("error out"=w170:errorcluster)  [unwired: 5 in, 1 out]
                                n143 = call <vilib>:"DB Tools Update Data.vi"("condition"=w172, "data"=w173, "error in (no error)"=w170, "columns"=w171, "table"="Code", "connection reference"=w175) -> ("error out"=w155:errorcluster)  [unwired: 4 in, 1 out]
                                n144 = call <vilib>:"Clear Errors.vi"("error in (no error)"=w155) -> ("error out"=w154:errorcluster)  [unwired: 5 in, 1 out]
                                n145 = call <vilib>:"Simple Error Handler.vi"("error in (no error)"=w154) -> ()  [unwired: 4 in, 5 out]
                              }
                              frame #2 {
                                n146 = call "GetSQLstring.vi"("联机模式"=w178) -> ("错误输出"=w190:errorcluster, "连接字符串"=w191:string)  [unwired: 9 in]
                                n147 = local read "CODE_ID 2"() -> (w181:string)
                                n148 = local read "CODE_ID"() -> (w182:string)
                                n149 = call-poly <vilib>:"DB Tools Open Connection.vi"("error in (no error)"=w190, "connection information"=w191) -> ("error out"=w185:errorcluster, "connection reference"=w186:T6)  [unwired: 6 in]
                                n150 = Concatenate Strings("WHERE CODE_ID =" ("condition"), w182) -> (w188:string)
                                n151 = call <vilib>:"Clear Errors.vi"("error in (no error)"=w185) -> ("error out"=w189:errorcluster)  [unwired: 5 in, 1 out]
                                n152 = Bundle("CODE_ID 2"=w181) -> (w187:cluster{"CODE_ID 2":string})  [unwired: 1 in]
                                n153 = call <vilib>:"DB Tools Update Data.vi"("condition"=w188, "data"=w187, "error in (no error)"=w189, "columns"=string[] ["CODE_ID"], "table"="Result\n", "connection reference"=w186) -> ("error out"=w179:errorcluster)  [unwired: 4 in, 1 out]
                                n154 = call <vilib>:"Simple Error Handler.vi"("error in (no error)"=w179) -> ()  [unwired: 4 in, 5 out]
                              }
                              frame #3 {
                                n155 = call "GetSQLstring.vi"("联机模式"=w192) -> ("错误输出"=w200:errorcluster, "连接字符串"=w199:string)  [unwired: 9 in]
                                n156 = local read "CODE_ID 2"() -> (w194:string)
                                n157 = local read "CODE_ID"() -> (w195:string)
                                n158 = call-poly <vilib>:"DB Tools Open Connection.vi"("error in (no error)"=w200, "connection information"=w199) -> ("error out"=w205:errorcluster, "connection reference"=w204:T6)  [unwired: 6 in]
                                n159 = Concatenate Strings("WHERE CODE_ID =" ("condition"), w195) -> (w202:string)
                                n160 = call <vilib>:"Clear Errors.vi"("error in (no error)"=w205) -> ("error out"=w201:errorcluster)  [unwired: 5 in, 1 out]
                                n161 = Bundle("CODE_ID 2"=w194) -> (w203:cluster{"CODE_ID 2":string})  [unwired: 1 in]
                                n162 = call <vilib>:"DB Tools Update Data.vi"("condition"=w202, "data"=w203, "error in (no error)"=w201, "columns"=string[] ["CODE_ID"], "table"="Test\n", "connection reference"=w204) -> ("error out"=w193:errorcluster)  [unwired: 4 in, 1 out]
                                n163 = call <vilib>:"Simple Error Handler.vi"("error in (no error)"=w193) -> ()  [unwired: 4 in, 5 out]
                              }
                            }
                          }
                          frame #1 {
                            w207 = string[] ["DEVICE_ID", "CODE_ID", "TEST_NAME", "TEST_VALUE", "TEST_VALUE_MIN", "TEST_VALUE_MAX", "TEST_VALUE_UNIT", "TEST_VALUE_RESULT"] ("columns")
                            w208 = "Test" ("table")
                            w213 = 0.0
                            n164 = local read "CODE_ID 2"() -> (w218:string)
                            n165 = local read "deviceid"() -> (w221:string)
                            n166 = Decimal String To Number(string=w221, default (0L)=i64 0 ("默认(0 I32)")) -> (number=w220:i64)  [unwired: 1 in, 1 out]
                            n167 = Decimal String To Number(string=w218, default (0L)=i64 0 ("默认(0 I32)")) -> (number=w219:i64)  [unwired: 1 in, 1 out]
                            n168 = call "GetSQLstring.vi"("联机模式"=w212) -> ("错误输出"=w224:errorcluster, "连接字符串"=w225:string)  [unwired: 9 in]
                            n169 = Bundle(w220, w219, "上下管柱安装合成结果", w213, w213, w213, "/", "OK") -> (w210:T7)  [unwired: 1 in]
                            n170 = call-poly <vilib>:"DB Tools Open Connection.vi"("error in (no error)"=w224, "connection information"=w225) -> ("error out"=w226:errorcluster, "connection reference"=w223:T6)  [unwired: 6 in]
                            n171 = call <vilib>:"DB Tools Insert Data.vi"("data"=w210, "error in (no error)"=w226, "columns"=w207, "table"=w208, "connection reference"=w223) -> ("error out"=w209:errorcluster, "connection reference out"=w206:T6)  [unwired: 5 in]
                            n172 = case shown="无错误" w209 {
                              selector: w209 -> [w227 w252]
                              tunnel: w207 -> [_ w249]
                              tunnel: w206 -> [w228 w235]
                              tunnel: w208 -> [_ w253]
                              tunnel: w210 -> [_ w244]
                              tunnel: [w228 w234] -> _
                              tunnel: [w227 w233] -> w222
                              frame No Error {
                              }
                              frame Error {
                                n173 = Delete From Array(array=w249, length=1 ("长度"), index=2 ("索引")) -> (array with subset deleted=w250:string[])  [unwired: 1 out]
                                n174 = Unbundle(w244) -> (w243:i64, w231:i64, w236:string, w242:dbl, w241:dbl, w240:dbl, w239:string, w238:string)
                                n175 = Bundle(w243, w231, w242, w241, w240, w239, w238) -> (w237:cluster{i64, i64, dbl, dbl, dbl, string, string})  [unwired: 1 in]
                                n176 = Number To Decimal String(number=w231) -> (decimal integer string=w230:string)  [unwired: 1 in]
                                n177 = call <vilib>:"Clear Errors.vi"("error in (no error)"=w252) -> ("error out"=w251:errorcluster)  [unwired: 5 in, 1 out]
                                n178 = Concatenate Strings("WHERE TEST_NAME ='" ("condition"), w236, "'", "AND CODE_ID =" ("condition"), w230) -> (w246:string)
                                n179 = call <vilib>:"DB Tools Update Data.vi"("condition"=w246, "data"=w237, "error in (no error)"=w251, "columns"=w250, "table"=w253, "connection reference"=w235) -> ("error out"=w233:errorcluster, "connection reference out"=w234:T6)  [unwired: 4 in]
                              }
                            }
                            n180 = call <vilib>:"Simple Error Handler.vi"("error in (no error)"=w222) -> ()  [unwired: 4 in, 5 out]
                          }
                          frame #2 {
                            n181 = shared-variable "我的电脑\\200滑移力曲线.lvlib\\备用_1"(u16 203 ("备用1")) -> ()  [unwired: 1 in, 1 out]
                          }
                        }
                      }
                    }
                  }
                  frame 203 {
                    n182 = global read "Global1.vi" "联机模式"() -> (w255:enum16{"单机", "追溯"})
                    n183 = case shown="\"追溯\"" w255 {
                      tunnel: w255 -> [_ w258]
                      frame "单机", Default {
                        n184 = shared-variable "我的电脑\\200滑移力曲线.lvlib\\备用_1"(u16 0 ("备用1")) -> ()  [unwired: 1 in, 1 out]
                        n185 = shared-variable "我的电脑\\200滑移力曲线.lvlib\\备用_3"(u16 0 ("备用1")) -> ()  [unwired: 1 in, 1 out]
                      }
                      frame "追溯" {
                        n186 = stacked-sequence {
                          tunnel: w258 -> [w259 _]
                          frame #0 {
                            n187 = Get Date/Time String(date format (0)=enum16{"short", "long", "abbreviated"}."short" ("日期格式(0)"), want seconds? (F)=FALSE ("需要秒？(F)")) -> (date string=w272:string, time string=w271:string)  [unwired: 1 in]
                            n188 = shared-variable "我的电脑\\200滑移力曲线.lvlib\\备用_8"() -> (w264:u16)  [unwired: 1 in, 1 out]
                            n189 = local read "CODE_ID 2"() -> (w277:string)
                            n190 = local read "deviceid"() -> (w280:string)
                            n191 = local read "USER_ID"() -> (w261:string)
                            n192 = case shown="2" w264 {
                              tunnel: ["" "OK" "NG"] -> w263
                              frame 0, Default {
                              }
                              frame 1 {
                              }
                              frame 2 {
                              }
                            }
                            n193 = Concatenate Strings(w272, " " ("字符串"), w271) -> (w268:string)
                            n194 = Decimal String To Number(string=w261, default (0L)=i64 0 ("默认(0 I32)")) -> (number=w260:i64)  [unwired: 1 in, 1 out]
                            n195 = Decimal String To Number(string=w277, default (0L)=i64 0 ("默认(0 I32)")) -> (number=w275:i64)  [unwired: 1 in, 1 out]
                            n196 = Decimal String To Number(string=w280, default (0L)=i64 0 ("默认(0 I32)")) -> (number=w278:i64)  [unwired: 1 in, 1 out]
                            n197 = Search and Replace String(replace all?=TRUE ("替换全部？(F)"), input string=w268, search string="/" ("替换字符串(\"\")"), replace string="-" ("替换字符串(\"\")")) -> (result string=w269:string)  [unwired: 4 in, 3 out]
                            n198 = Bundle(w278, w260, w275, w263, "result string"=w269) -> (w282:T8)  [unwired: 1 in]
                            n199 = call "GetSQLstring.vi"("联机模式"=w259) -> ("错误输出"=w285:errorcluster, "连接字符串"=w286:string)  [unwired: 9 in]
                            n200 = Build Array(w282) -> (w281:T9)
                            n201 = call-poly <vilib>:"DB Tools Open Connection.vi"("error in (no error)"=w285, "connection information"=w286) -> ("error out"=w287:errorcluster, "connection reference"=w284:T6)  [unwired: 6 in]
                            n202 = for {
                              tunnel: w281 -> [w295] mode=indexing
                              tunnel: w284 -> [w293]
                              shift-right: [w291] -> w283
                              shift-left: w287 -> [w298]
                              w294 = string[] ["DEVICE_ID", "USER_ID", "CODE_ID", "RESULT_VALUE", "RESULT_TIME"] ("columns")
                              w296 = "Result" ("table")
                              n203 = call <vilib>:"DB Tools Insert Data.vi"("data"=w295, "error in (no error)"=w298, "columns"=w294, "table"=w296, "connection reference"=w293) -> ("error out"=w297:errorcluster, "connection reference out"=w292:T6)  [unwired: 5 in]
                              n204 = case shown="错误" w297 {
                                selector: w297 -> [w299 w320]
                                tunnel: w294 -> [_ w317]
                                tunnel: w292 -> [w300 w309]
                                tunnel: w296 -> [_ w321]
                                tunnel: w295 -> [_ w313]
                                tunnel: [w300 w308] -> _
                                tunnel: [w299 w307] -> w291
                                frame No Error {
                                }
                                frame Error {
                                n205 = Array Subset(array=w317, index=3 ("长度"), length=2 ("索引")) -> (w318:string[])
                                n206 = Unbundle(w313) -> (w302:i64, w305:i64, w312:string, "result string"=w311:string)  [unwired: 1 out]
                                n207 = Number To Decimal String(number=w302) -> (decimal integer string=w301:string)  [unwired: 1 in]
                                n208 = Number To Decimal String(number=w305) -> (decimal integer string=w306:string)  [unwired: 1 in]
                                n209 = Concatenate Strings("WHERE CODE_ID =" ("condition"), w306, "AND DEVICE_ID =", w301) -> (w314:string)
                                n210 = Bundle(w312, "result string"=w311) -> (w310:cluster{string, "result string":string})  [unwired: 1 in]
                                n211 = call <vilib>:"Clear Errors.vi"("error in (no error)"=w320) -> ("error out"=w319:errorcluster)  [unwired: 5 in, 1 out]
                                n212 = call <vilib>:"DB Tools Update Data.vi"("condition"=w314, "data"=w310, "error in (no error)"=w319, "columns"=w318, "table"=w321, "connection reference"=w309) -> ("error out"=w307:errorcluster, "connection reference out"=w308:T6)  [unwired: 4 in]
                                }
                              }
                            }
                            n213 = call <vilib>:"Simple Error Handler.vi"("error in (no error)"=w283) -> ()  [unwired: 4 in, 5 out]
                          }
                          frame #1 {
                            n214 = shared-variable "我的电脑\\200滑移力曲线.lvlib\\备用_1"(u16 0 ("备用1")) -> ()  [unwired: 1 in, 1 out]
                            n215 = shared-variable "我的电脑\\200滑移力曲线.lvlib\\备用_3"(u16 0 ("备用1")) -> ()  [unwired: 1 in, 1 out]
                          }
                        }
                      }
                    }
                  }
                  frame 100 {
                    n216 = stacked-sequence {
                      frame #0 {
                        n217 = control-ref of="滑移力复检曲线"() -> (w329:refnum<vi>)
                        n218 = Wait (ms)(milliseconds to wait=u32 100 ("等待时间（毫秒）")) -> ()  [unwired: 1 out]
                        n219 = local read "滑移力复检曲线"() -> (w328:cluster{dbl[], dbl[]}[])
                        n220 = global read "Global.vi" "判定参数"() -> (w326:T10)
                        n221 = global write "A131258.vi" "滑移力位移曲线"(w329) -> ()
                        n222 = global read "Global.vi" "Result"() -> (w327:refnum<vi>)
                        n223 = call "滑移力复测判定.vi"("压力判定项"="压力判定项", "拉力判定项"="判定项", "滑移力曲线"=w328) -> ()  [unwired: 8 in, 1 out]
                        n224 = call "复检判定.vi"("Result"=w327, "判定参数"=w326, "XY曲线"=w328) -> ("OK？"=w325:bool)  [unwired: 8 in]
                        n225 = case shown="假" w325 {
                          tunnel: [2 1] -> w324
                          frame False {
                          }
                          frame True {
                          }
                        }
                        n226 = disable-structure shown="禁用" {
                          frame Disabled {
                            n227 = Build Array "创建数组"("OK") -> (w336:string[])
                            n228 = Build Array "创建数组"(w336) -> (w337:string[][])
                            n229 = local write "管柱合成报表"(w337) -> ()
                          }
                          frame Enabled {
                          }
                        }
                        n230 = shared-variable "我的电脑\\200滑移力曲线.lvlib\\备用_2"(w324) -> ()  [unwired: 1 in, 1 out]
                      }
                      frame #1 {
                        w405 = i16 3 ("精度(6)")
                        n231 = local read "判定"() -> (w410:string[][])
                        n232 = Index Array(array=w410) -> (element #1=w409:string[], element #2=w399:string[], element #3=w392:string[])  [unwired: 12 in, 3 out]
                        n233 = Index Array(array=w409) -> (element #1=w408:string, element #2=w407:string, element #3=w406:string)  [unwired: 3 in]
                        n234 = Index Array(array=w392) -> (element #1=w391:string, element #2=w390:string, element #3=w389:string)  [unwired: 3 in]
                        n235 = Index Array(array=w399) -> (element #1=w398:string, element #2=w397:string, element #3=w396:string)  [unwired: 3 in]
                        n236 = Fract/Exp String To Number(string=w391) -> (number=w386:dbl)  [unwired: 3 in, 1 out]
                        n237 = Fract/Exp String To Number(string=w390) -> (number=w388:dbl)  [unwired: 3 in, 1 out]
                        n238 = Fract/Exp String To Number(string=w389) -> (number=w387:dbl)  [unwired: 3 in, 1 out]
                        n239 = Fract/Exp String To Number(string=w408) -> (number=w401:dbl)  [unwired: 3 in, 1 out]
                        n240 = Fract/Exp String To Number(string=w407) -> (number=w400:dbl)  [unwired: 3 in, 1 out]
                        n241 = Fract/Exp String To Number(string=w406) -> (number=w402:dbl)  [unwired: 3 in, 1 out]
                        n242 = Fract/Exp String To Number(string=w398) -> (number=w393:dbl)  [unwired: 3 in, 1 out]
                        n243 = Fract/Exp String To Number(string=w397) -> (number=w395:dbl)  [unwired: 3 in, 1 out]
                        n244 = Fract/Exp String To Number(string=w396) -> (number=w394:dbl)  [unwired: 3 in, 1 out]
                        n245 = In Range and Coerce(upper limit=w387, x=w388, lower limit=w386) -> (In Range?=w343:bool)  [unwired: 1 out]
                        n246 = In Range and Coerce(upper limit=w402, x=w400, lower limit=w401) -> (In Range?=w345:bool)  [unwired: 1 out]
                        n247 = case shown="真" w345 {
                          tunnel: ["NG" "OK"] -> w423
                          frame False {
                          }
                          frame True {
                          }
                        }
                        n248 = case shown="真" w343 {
                          tunnel: ["NG" "OK"] -> w414
                          frame False {
                          }
                          frame True {
                          }
                        }
                        n249 = In Range and Coerce(upper limit=w394, x=w395, lower limit=w393) -> (In Range?=w344:bool)  [unwired: 1 out]
                        n250 = Number To Fractional String(number=w386) -> (F-format string=w417:string)  [unwired: 3 in]
                        n251 = Number To Fractional String ("数值至小数字符串转换")(number=w388) -> (F-format string=w416:string)  [unwired: 3 in]
                        n252 = Number To Fractional String(number=w387) -> (F-format string=w415:string)  [unwired: 3 in]
                        n253 = case shown="真" w344 {
                          tunnel: ["NG" "OK"] -> w418
                          frame False {
                          }
                          frame True {
                          }
                        }
                        n254 = Number To Fractional String ("数值至小数字符串转换")(number=w401, precision (6)=w405) -> (F-format string=w422:string)  [unwired: 2 in]
                        n255 = Number To Fractional String ("数值至小数字符串转换")(number=w400, precision (6)=w405) -> (F-format string=w404:string)  [unwired: 2 in]
                        n256 = Number To Fractional String ("数值至小数字符串转换")(number=w402, precision (6)=w405) -> (F-format string=w403:string)  [unwired: 2 in]
                        n257 = Number To Fractional String(number=w393) -> (F-format string=w421:string)  [unwired: 3 in]
                        n258 = Number To Fractional String(number=w395) -> (F-format string=w420:string)  [unwired: 3 in]
                        n259 = Number To Fractional String(number=w394) -> (F-format string=w419:string)  [unwired: 3 in]
                        n260 = Build Array(w417, w416, w415, w414) -> (w411:string[])
                        n261 = local read "判定"() -> (w385:string[][])
                        n262 = Build Array(w421, w420, w419, w418) -> (w412:string[])
                        n263 = Build Array(w422, w404, w403, w423) -> (w413:string[])
                        n264 = Index Array(array=w385, index (row) #1=3 ("索引 (行)")) -> (element #1=w383:string[], element #2=w371:string[], element #3=w364:string[])  [unwired: 5 in]
                        n265 = Index Array(array=w383) -> (element #1=w382:string, element #2=w381:string, element #3=w380:string)  [unwired: 3 in]
                        n266 = Index Array(array=w371) -> (element #1=w370:string, element #2=w369:string, element #3=w368:string)  [unwired: 3 in]
                        n267 = Index Array(array=w364) -> (element #1=w363:string, element #2=w362:string, element #3=w361:string)  [unwired: 3 in]
                        n268 = Fract/Exp String To Number(string=w382) -> (number=w377:dbl)  [unwired: 3 in, 1 out]
                        n269 = Fract/Exp String To Number(string=w381) -> (number=w379:dbl)  [unwired: 3 in, 1 out]
                        n270 = Fract/Exp String To Number(string=w380) -> (number=w378:dbl)  [unwired: 3 in, 1 out]
                        n271 = Fract/Exp String To Number(string=w370) -> (number=w365:dbl)  [unwired: 3 in, 1 out]
                        n272 = Fract/Exp String To Number(string=w369) -> (number=w367:dbl)  [unwired: 3 in, 1 out]
                        n273 = Fract/Exp String To Number(string=w368) -> (number=w366:dbl)  [unwired: 3 in, 1 out]
                        n274 = Fract/Exp String To Number(string=w363) -> (number=w358:dbl)  [unwired: 3 in, 1 out]
                        n275 = Fract/Exp String To Number(string=w362) -> (number=w360:dbl)  [unwired: 3 in, 1 out]
                        n276 = Fract/Exp String To Number(string=w361) -> (number=w359:dbl)  [unwired: 3 in, 1 out]
                        n277 = In Range and Coerce(upper limit=w378, x=w379, lower limit=w377) -> (In Range?=w342:bool)  [unwired: 1 out]
                        n278 = In Range and Coerce(upper limit=w366, x=w367, lower limit=w365) -> (In Range?=w341:bool)  [unwired: 1 out]
                        n279 = In Range and Coerce(upper limit=w359, x=w360, lower limit=w358) -> (In Range?=w340:bool)  [unwired: 1 out]
                        n280 = Compound Arithmetic op=AND ("复合运算")(w345, w344, w343, w342, w341, w340) -> (w339:bool)
                        n281 = Not(x=w339) -> (.not. x?=w346:bool)
                        n282 = Build Array(w339, w346) -> (w347:bool[])
                        n283 = Boolean Array To Number ("布尔数组至数值转换")(Boolean array=w347) -> ()  [unwired: 1 out]
                        n284 = Number To Fractional String(number=w377) -> (F-format string=w376:string)  [unwired: 3 in]
                        n285 = Number To Fractional String ("数值至小数字符串转换")(number=w379) -> (F-format string=w375:string)  [unwired: 3 in]
                        n286 = Number To Fractional String(number=w365) -> (F-format string=w357:string)  [unwired: 3 in]
                        n287 = Number To Fractional String(number=w378) -> (F-format string=w374:string)  [unwired: 3 in]
                        n288 = case shown="真" w342 {
                          tunnel: ["NG" "OK"] -> w373
                          frame False {
                          }
                          frame True {
                          }
                        }
                        n289 = Number To Fractional String ("数值至小数字符串转换")(number=w367) -> (F-format string=w356:string)  [unwired: 3 in]
                        n290 = Number To Fractional String(number=w366) -> (F-format string=w355:string)  [unwired: 3 in]
                        n291 = case shown="真" w341 {
                          tunnel: ["NG" "OK"] -> w354
                          frame False {
                          }
                          frame True {
                          }
                        }
                        n292 = Number To Fractional String(number=w358) -> (F-format string=w353:string)  [unwired: 3 in]
                        n293 = Number To Fractional String ("数值至小数字符串转换")(number=w360) -> (F-format string=w352:string)  [unwired: 3 in]
                        n294 = Number To Fractional String(number=w359) -> (F-format string=w351:string)  [unwired: 3 in]
                        n295 = case shown="假" w340 {
                          tunnel: ["NG" "OK"] -> w350
                          frame False {
                          }
                          frame True {
                          }
                        }
                        n296 = Build Array(w376, w375, w374, w373) -> (w372:string[])
                        n297 = Build Array(w357, w356, w355, w354) -> (w349:string[])
                        n298 = Build Array(w353, w352, w351, w350) -> (w348:string[])
                        n299 = local read "表格控件"() -> (w338:string[][])
                        n300 = Build Array(w413, w412, w411, w372, w349, w348) -> ()  [unwired: 1 out]
                        n301 = local write "管柱合成报表"(w338) -> ()
                      }
                      frame #2 {
                        n302 = shared-variable "我的电脑\\200滑移力曲线.lvlib\\备用_3"(u16 1 ("备用1")) -> ()  [unwired: 1 in, 1 out]
                        n303 = Wait (ms)(milliseconds to wait=u32 500 ("等待时间（毫秒）")) -> ()  [unwired: 1 out]
                        n304 = shared-variable "我的电脑\\200滑移力曲线.lvlib\\备用_1"(u16 101 ("备用1")) -> ()  [unwired: 1 in, 1 out]
                        n305 = shared-variable "我的电脑\\200滑移力曲线.lvlib\\备用_2"() -> (w437:u16)  [unwired: 1 in, 1 out]
                        n306 = control-ref of="管柱合成报表"() -> (w439:refnum<vi>)
                        n307 = call "浮动通知.vi"("通知内容"="报表生成中" ("Status")) -> ()  [unwired: 11 in]
                        n308 = case shown="2" w437 {
                          frame 0, Default {
                          }
                          frame 1 {
                            n309 = local write "合格指示灯"(TRUE ("合格指示灯")) -> ()
                            n310 = local write "不合格指示灯"(FALSE ("不合格指示灯")) -> ()
                            n311 = local write "滑移力判定结果"(bool[][] [[TRUE, TRUE]] ("判定结果")) -> ()
                            n312 = local write "装配结果"("合格" ("文本.文本")) -> ()
                            n313 = property on="装配结果" class="Str"("Text.BGColor"=u32 6618880 ("文本.文本颜色:背景色")) -> ()  [unwired: 2 in, 2 out]
                          }
                          frame 2 {
                            n314 = local write "滑移力判定结果"(bool[][] [[TRUE, FALSE]] ("判定结果")) -> ()
                            n315 = property on="装配结果" class="Str"("Text.BGColor"=u32 16711680 ("文本.文本颜色:背景色")) -> ()  [unwired: 2 in, 2 out]
                            n316 = local write "装配结果"("不合格" ("文本.文本")) -> ()
                            "合格指示灯" <- FALSE ("合格指示灯")
                            "不合格指示灯" <- TRUE ("不合格指示灯")
                          }
                        }
                        n317 = global write "Global.vi" "滑移力报表"(w439) -> ()
                      }
                    }
                  }
                  frame 101 {
                    n318 = shared-variable "我的电脑\\200滑移力曲线.lvlib\\备用_1"(u16 102 ("备用1")) -> ()  [unwired: 1 in, 1 out]
                    n319 = Wait (ms)(milliseconds to wait=u32 800 ("等待时间（毫秒）")) -> ()  [unwired: 1 out]
                    n320 = shared-variable "我的电脑\\Global.lvlib\\工位追溯码"() -> (w452:string)  [unwired: 1 in, 1 out]
                    n321 = shared-variable "我的电脑\\Global.lvlib\\传感器码"() -> (w453:string)  [unwired: 1 in, 1 out]
                    n322 = Concatenate Strings(w453, "；" ("字符串"), w452) -> (w454:string)
                    n323 = call "Report_A131258.vi"("文件重命名"=TRUE, "文件名称"=w454, "布尔数组"="滑移力判定结果") -> ()  [unwired: 8 in, 1 out]
                  }
                  frame 102 {
                    n324 = global read "Global1.vi" "联机模式"() -> (w460:enum16{"单机", "追溯"})
                    n325 = case shown="\"追溯\"" w460 {
                      tunnel: w460 -> [_ w462]
                      frame "单机", Default {
                        n326 = shared-variable "我的电脑\\200滑移力曲线.lvlib\\备用_1"(u16 103 ("备用1")) -> ()  [unwired: 1 in, 1 out]
                      }
                      frame "追溯" {
                        n327 = stacked-sequence {
                          tunnel: w462 -> [w463 w594 _]
                          frame #0 {
                            n328 = stacked-sequence {
                              tunnel: w463 -> [w464 w478 w496 w506]
                              frame #0 {
                                n329 = call "GetSQLstring.vi"("联机模式"=w464) -> ("错误输出"=w476:errorcluster, "连接字符串"=w477:string)  [unwired: 9 in]
                                n330 = call-poly <vilib>:"DB Tools Open Connection.vi"("error in (no error)"=w476, "connection information"=w477) -> ("error out"=w471:errorcluster, "connection reference"=w472:T6)  [unwired: 6 in]
                                n331 = local read "CODE_ID 2"() -> (w467:string)
                                n332 = local read "CODE_ID"() -> (w468:string)
                                n333 = Concatenate Strings("WHERE CODE_ID =" ("condition"), w468) -> (w474:string)
                                n334 = Bundle("CODE_ID 2"=w467) -> (w473:cluster{"CODE_ID 2":string})  [unwired: 1 in]
                                n335 = call <vilib>:"Clear Errors.vi"("error in (no error)"=w471) -> ("error out"=w475:errorcluster)  [unwired: 5 in, 1 out]
                                n336 = call <vilib>:"DB Tools Update Data.vi"("condition"=w474, "data"=w473, "error in (no error)"=w475, "columns"=string[] ["CODE_ID"], "table"="Result\n", "connection reference"=w472) -> ("error out"=w465:errorcluster)  [unwired: 4 in, 1 out]
                                n337 = call <vilib>:"Simple Error Handler.vi"("error in (no error)"=w465) -> ()  [unwired: 4 in, 5 out]
                              }
                              frame #1 {
                                n338 = call "GetSQLstring.vi"("联机模式"=w478) -> ("错误输出"=w486:errorcluster, "连接字符串"=w485:string)  [unwired: 9 in]
                                n339 = call-poly <vilib>:"DB Tools Open Connection.vi"("error in (no error)"=w486, "connection information"=w485) -> ("error out"=w491:errorcluster, "connection reference"=w490:T6)  [unwired: 6 in]
                                n340 = local read "CODE_ID 2"() -> (w480:string)
                                n341 = local read "CODE_ID"() -> (w481:string)
                                n342 = Concatenate Strings("WHERE CODE_ID =" ("condition"), w481) -> (w488:string)
                                n343 = Bundle("CODE_ID 2"=w480) -> (w489:cluster{"CODE_ID 2":string})  [unwired: 1 in]
                                n344 = call <vilib>:"Clear Errors.vi"("error in (no error)"=w491) -> ("error out"=w487:errorcluster)  [unwired: 5 in, 1 out]
                                n345 = call <vilib>:"DB Tools Update Data.vi"("condition"=w488, "data"=w489, "error in (no error)"=w487, "columns"=string[] ["CODE_ID"], "table"="Test\n", "connection reference"=w490) -> ("error out"=w479:errorcluster)  [unwired: 4 in, 1 out]
                                n346 = call <vilib>:"Simple Error Handler.vi"("error in (no error)"=w479) -> ()  [unwired: 4 in, 5 out]
                              }
                              frame #2 {
                                n347 = local read "CODE_ID"() -> (w502:string)
                                n348 = call "GetSQLstring.vi"("联机模式"=w496) -> ("错误输出"=w498:errorcluster, "连接字符串"=w497:string)  [unwired: 9 in]
                                n349 = Concatenate Strings("WHERE CODE_ID =" ("condition"), w502) -> (w501:string)
                                n350 = call-poly <vilib>:"DB Tools Open Connection.vi"("error in (no error)"=w498, "connection information"=w497) -> ("error out"=w494:errorcluster, "connection reference"=w495:T6)  [unwired: 6 in]
                                n351 = call <vilib>:"DB Tools Delete Data.vi"("condition"=w501, "error in (no error)"=w494, "table"="Code", "connection reference"=w495) -> ("error out"=w493:errorcluster)  [unwired: 6 in, 1 out]
                                n352 = call <vilib>:"Clear Errors.vi"("error in (no error)"=w493) -> ("error out"=w492:errorcluster)  [unwired: 5 in, 1 out]
                                n353 = call <vilib>:"Simple Error Handler.vi"("error in (no error)"=w492) -> ()  [unwired: 4 in, 5 out]
                              }
                              frame #3 {
                                n354 = local read "productid"() -> (w517:string)
                                n355 = shared-variable "我的电脑\\Global.lvlib\\工位追溯码"() -> (w515:string)  [unwired: 1 in, 1 out]
                                n356 = Decimal String To Number(string=w517, default (0L)=i64 0 ("默认(0 I32)")) -> (number=w518:i64)  [unwired: 1 in, 1 out]
                                n357 = local read "产品条码"() -> (w503:string)
                                n358 = Bundle(w518, "String"=w515, "产品条码"=w503) -> (w516:cluster{i64, "String":string, "产品条码":string})  [unwired: 1 in]
                                n359 = call "GetSQLstring.vi"("联机模式"=w506) -> ("错误输出"=w514:errorcluster, "连接字符串"=w513:string)  [unwired: 9 in]
                                n360 = local read "CODE_ID 2"() -> (w526:string)
                                n361 = Unbundle(w516) -> ("产品条码"=w523:string)  [unwired: 2 out]
                                n362 = call-poly <vilib>:"DB Tools Open Connection.vi"("error in (no error)"=w514, "connection information"=w513) -> ("error out"=w525:errorcluster, "connection reference"=w524:T6)  [unwired: 6 in]
                                n363 = Concatenate Strings("WHERE CODE_ID =" ("condition"), w526) -> (w521:string)
                                n364 = call <vilib>:"Clear Errors.vi"("error in (no error)"=w525) -> ("error out"=w519:errorcluster)  [unwired: 5 in, 1 out]
                                n365 = Bundle("产品条码"=w523) -> (w522:cluster{"产品条码":string})  [unwired: 1 in]
                                n366 = Array Subset(array=string[] ["PRODUCT_ID", "CODE_MAIN", "CODE_SENSOR"] ("columns"), index=2 ("长度"), length=1 ("索引")) -> (w520:string[])
                                n367 = call <vilib>:"DB Tools Update Data.vi"("condition"=w521, "data"=w522, "error in (no error)"=w519, "columns"=w520, "table"="Code", "connection reference"=w524) -> ("error out"=w505:errorcluster)  [unwired: 4 in, 1 out]
                                n368 = call <vilib>:"Clear Errors.vi"("error in (no error)"=w505) -> ("error out"=w504:errorcluster)  [unwired: 5 in, 1 out]
                                n369 = call <vilib>:"Simple Error Handler.vi"("error in (no error)"=w504) -> ()  [unwired: 4 in, 5 out]
                              }
                            }
                          }
                          frame #1 {
                            w541 = "N"
                            n370 = shared-variable "我的电脑\\200滑移力曲线.lvlib\\备用_2"() -> (w572:u16)  [unwired: 1 in, 1 out]
                            n371 = local read "判定"() -> (w593:string[][])
                            n372 = case shown="2" w572 {
                              tunnel: ["" "OK" "NG"] -> w540
                              frame 0, Default {
                              }
                              frame 1 {
                              }
                              frame 2 {
                              }
                            }
                            n373 = local read "CODE_ID 2"() -> (w582:string)
                            n374 = local read "deviceid"() -> (w584:string)
                            n375 = Index Array(array=w593, index (row) #1=0 ("索引 (行)"), index (row) #2=1 ("索引 (行)"), index (row) #3=4 ("索引 (行)"), index (row) #4=0 ("索引 (行)")) -> (element #1=w592:string[], element #2=w568:string[], element #3=w558:string[], element #4=w539:string[])  [unwired: 4 in]
                            n376 = Index Array(array=w539, index #1=1 ("索引"), index #2=0 ("索引"), index #3=2 ("索引")) -> (element #1=w534:string, element #2=w533:string, element #3=w532:string)
                            n377 = Index Array(array=w558, index #1=1 ("索引"), index #2=0 ("索引"), index #3=2 ("索引")) -> (element #1=w556:string, element #2=w555:string, element #3=w554:string)
                            n378 = Index Array(array=w568, index #1=1 ("索引"), index #2=0 ("索引"), index #3=2 ("索引")) -> (element #1=w571:string, element #2=w570:string, element #3=w569:string)
                            n379 = Index Array(array=w592, index #1=1 ("索引"), index #2=0 ("索引"), index #3=2 ("索引")) -> (element #1=w590:string, element #2=w578:string, element #3=w577:string)
                            n380 = Decimal String To Number(string=w584, default (0L)=i64 0 ("默认(0 I32)")) -> (number=w547:i64)  [unwired: 1 in, 1 out]
                            n381 = Decimal String To Number(string=w582, default (0L)=i64 0 ("默认(0 I32)")) -> (number=w546:i64)  [unwired: 1 in, 1 out]
                            n382 = Fract/Exp String To Number(string=w590) -> (number=w579:dbl)  [unwired: 3 in, 1 out]
                            n383 = Fract/Exp String To Number(string=w578) -> (number=w576:dbl)  [unwired: 3 in, 1 out]
                            n384 = Fract/Exp String To Number(string=w577) -> (number=w575:dbl)  [unwired: 3 in, 1 out]
                            n385 = Fract/Exp String To Number(string=w571) -> (number=w563:dbl)  [unwired: 3 in, 1 out]
                            n386 = Fract/Exp String To Number(string=w570) -> (number=w562:dbl)  [unwired: 3 in, 1 out]
                            n387 = Fract/Exp String To Number(string=w569) -> (number=w561:dbl)  [unwired: 3 in, 1 out]
                            n388 = Fract/Exp String To Number(string=w556) -> (number=w553:dbl)  [unwired: 3 in, 1 out]
                            n389 = Fract/Exp String To Number(string=w555) -> (number=w552:dbl)  [unwired: 3 in, 1 out]
                            n390 = Fract/Exp String To Number(string=w554) -> (number=w551:dbl)  [unwired: 3 in, 1 out]
                            n391 = Fract/Exp String To Number(string=w534) -> (number=w544:dbl)  [unwired: 3 in, 1 out]
                            n392 = Fract/Exp String To Number(string=w533) -> (number=w543:dbl)  [unwired: 3 in, 1 out]
                            n393 = Fract/Exp String To Number(string=w532) -> (number=w542:dbl)  [unwired: 3 in, 1 out]
                            n394 = Bundle(w547, w546, "拉力最小值", w563, w562, w561, w541, w540) -> (w531:T7)  [unwired: 1 in]
                            n395 = Bundle(w547, w546, "拉力最大值", w579, w576, w575, w541, w540) -> (w528:T7)  [unwired: 1 in]
                            n396 = Bundle(w547, w546, "压力最大值", w553, w552, w551, w541, w540) -> (w530:T7)  [unwired: 1 in]
                            n397 = Bundle(w547, w546, "压力最小值", w544, w543, w542, w541, w540) -> (w529:T7)  [unwired: 1 in]
                            n398 = call "GetSQLstring.vi"("联机模式"=w594) -> ("错误输出"=w587:errorcluster, "连接字符串"=w588:string)  [unwired: 9 in]
                            n399 = Build Array(w528, w531, w530, w529) -> (w527:T11)
                            n400 = call-poly <vilib>:"DB Tools Open Connection.vi"("error in (no error)"=w587, "connection information"=w588) -> ("error out"=w589:errorcluster, "connection reference"=w586:T6)  [unwired: 6 in]
                            n401 = for {
                              tunnel: w589 -> [w602]
                              tunnel: w586 -> [w601]
                              tunnel: w527 -> [w595] mode=indexing
                              w598 = string[] ["DEVICE_ID", "CODE_ID", "TEST_NAME", "TEST_VALUE", "TEST_VALUE_MIN", "TEST_VALUE_MAX", "TEST_VALUE_UNIT", "TEST_VALUE_RESULT"] ("columns")
                              w596 = "Test" ("table")
                              n402 = call <vilib>:"DB Tools Insert Data.vi"("data"=w595, "error in (no error)"=w602, "columns"=w598, "table"=w596, "connection reference"=w601) -> ("error out"=w599:errorcluster, "connection reference out"=w597:T6)  [unwired: 5 in]
                              n403 = case shown="错误" w599 {
                                selector: w599 -> [w603 w628]
                                tunnel: w598 -> [_ w625]
                                tunnel: w597 -> [w604 w610]
                                tunnel: w596 -> [_ w629]
                                tunnel: w595 -> [_ w619]
                                tunnel: [w604 w609] -> _
                                tunnel: [w603 w608] -> w600
                                frame No Error {
                                }
                                frame Error {
                                n404 = Delete From Array(array=w625, length=1 ("长度"), index=2 ("索引")) -> (array with subset deleted=w626:string[])  [unwired: 1 out]
                                n405 = Unbundle(w619) -> (w618:i64, w606:i64, w611:string, w617:dbl, w616:dbl, w615:dbl, w614:string, w613:string)
                                n406 = Number To Decimal String(number=w606) -> (decimal integer string=w605:string)  [unwired: 1 in]
                                n407 = Bundle(w618, w606, w617, w616, w615, w614, w613) -> (w612:cluster{i64, i64, dbl, dbl, dbl, string, string})  [unwired: 1 in]
                                n408 = call <vilib>:"Clear Errors.vi"("error in (no error)"=w628) -> ("error out"=w627:errorcluster)  [unwired: 5 in, 1 out]
                                n409 = Concatenate Strings("WHERE TEST_NAME ='" ("condition"), w611, "'", "AND CODE_ID =" ("condition"), w605) -> (w621:string)
                                n410 = call <vilib>:"DB Tools Update Data.vi"("condition"=w621, "data"=w612, "error in (no error)"=w627, "columns"=w626, "table"=w629, "connection reference"=w610) -> ("error out"=w608:errorcluster, "connection reference out"=w609:T6)  [unwired: 4 in]
                                }
                              }
                              n411 = call <vilib>:"Simple Error Handler.vi"("error in (no error)"=w600) -> ()  [unwired: 4 in, 5 out]
                            }
                          }
                          frame #2 {
                            n412 = shared-variable "我的电脑\\200滑移力曲线.lvlib\\备用_1"(u16 103 ("备用1")) -> ()  [unwired: 1 in, 1 out]
                          }
                        }
                      }
                    }
                  }
                  frame 103 {
                    n413 = global read "Global1.vi" "联机模式"() -> (w634:enum16{"单机", "追溯"})
                    n414 = case shown="\"追溯\"" w634 {
                      tunnel: w634 -> [_ w637]
                      frame "单机", Default {
                        n415 = shared-variable "我的电脑\\200滑移力曲线.lvlib\\备用_1"(u16 0 ("备用1")) -> ()  [unwired: 1 in, 1 out]
                        n416 = shared-variable "我的电脑\\200滑移力曲线.lvlib\\备用_3"(u16 0 ("备用1")) -> ()  [unwired: 1 in, 1 out]
                      }
                      frame "追溯" {
                        n417 = stacked-sequence {
                          tunnel: w637 -> [w638 _]
                          frame #0 {
                            n418 = Get Date/Time String(date format (0)=enum16{"short", "long", "abbreviated"}."short" ("日期格式(0)"), want seconds? (F)=FALSE ("需要秒？(F)")) -> (date string=w651:string, time string=w650:string)  [unwired: 1 in]
                            n419 = shared-variable "我的电脑\\200滑移力曲线.lvlib\\备用_2"() -> (w643:u16)  [unwired: 1 in, 1 out]
                            n420 = local read "CODE_ID 2"() -> (w656:string)
                            n421 = local read "deviceid"() -> (w659:string)
                            n422 = local read "USER_ID"() -> (w640:string)
                            n423 = case shown="2" w643 {
                              tunnel: ["" "OK" "NG"] -> w642
                              frame 0, Default {
                              }
                              frame 1 {
                              }
                              frame 2 {
                              }
                            }
                            n424 = Concatenate Strings(w651, " " ("字符串"), w650) -> (w647:string)
                            n425 = Decimal String To Number(string=w640, default (0L)=i64 0 ("默认(0 I32)")) -> (number=w639:i64)  [unwired: 1 in, 1 out]
                            n426 = Decimal String To Number(string=w656, default (0L)=i64 0 ("默认(0 I32)")) -> (number=w654:i64)  [unwired: 1 in, 1 out]
                            n427 = Decimal String To Number(string=w659, default (0L)=i64 0 ("默认(0 I32)")) -> (number=w657:i64)  [unwired: 1 in, 1 out]
                            n428 = Search and Replace String(replace all?=TRUE ("替换全部？(F)"), input string=w647, search string="/" ("替换字符串(\"\")"), replace string="-" ("替换字符串(\"\")")) -> (result string=w648:string)  [unwired: 4 in, 3 out]
                            n429 = Bundle(w657, w639, w654, w642, "result string"=w648) -> (w661:T8)  [unwired: 1 in]
                            n430 = call "GetSQLstring.vi"("联机模式"=w638) -> ("错误输出"=w664:errorcluster, "连接字符串"=w665:string)  [unwired: 9 in]
                            n431 = Build Array(w661) -> (w660:T9)
                            n432 = call-poly <vilib>:"DB Tools Open Connection.vi"("error in (no error)"=w664, "connection information"=w665) -> ("error out"=w666:errorcluster, "connection reference"=w663:T6)  [unwired: 6 in]
                            n433 = for {
                              tunnel: w660 -> [w674] mode=indexing
                              tunnel: w663 -> [w672]
                              shift-right: [w670] -> w662
                              shift-left: w666 -> [w677]
                              w673 = string[] ["DEVICE_ID", "USER_ID", "CODE_ID", "RESULT_VALUE", "RESULT_TIME"] ("columns")
                              w675 = "Result" ("table")
                              n434 = call <vilib>:"DB Tools Insert Data.vi"("data"=w674, "error in (no error)"=w677, "columns"=w673, "table"=w675, "connection reference"=w672) -> ("error out"=w676:errorcluster, "connection reference out"=w671:T6)  [unwired: 5 in]
                              n435 = case shown="错误" w676 {
                                selector: w676 -> [w678 w699]
                                tunnel: w673 -> [_ w696]
                                tunnel: w671 -> [w679 w688]
                                tunnel: w675 -> [_ w700]
                                tunnel: w674 -> [_ w692]
                                tunnel: [w679 w687] -> _
                                tunnel: [w678 w686] -> w670
                                frame No Error {
                                }
                                frame Error {
                                n436 = Array Subset(array=w696, index=3 ("长度"), length=2 ("索引")) -> (w697:string[])
                                n437 = Unbundle(w692) -> (w682:i64, w684:i64, w691:string, "result string"=w690:string)  [unwired: 1 out]
                                n438 = Number To Decimal String(number=w682) -> (decimal integer string=w681:string)  [unwired: 1 in]
                                n439 = Number To Decimal String(number=w684) -> (decimal integer string=w685:string)  [unwired: 1 in]
                                n440 = Concatenate Strings("WHERE CODE_ID =" ("condition"), w685, "AND DEVICE_ID =", w681) -> (w693:string)
                                n441 = Bundle(w691, "result string"=w690) -> (w689:cluster{string, "result string":string})  [unwired: 1 in]
                                n442 = call <vilib>:"Clear Errors.vi"("error in (no error)"=w699) -> ("error out"=w698:errorcluster)  [unwired: 5 in, 1 out]
                                n443 = call <vilib>:"DB Tools Update Data.vi"("condition"=w693, "data"=w689, "error in (no error)"=w698, "columns"=w697, "table"=w700, "connection reference"=w688) -> ("error out"=w686:errorcluster, "connection reference out"=w687:T6)  [unwired: 4 in]
                                }
                              }
                            }
                            n444 = call <vilib>:"Simple Error Handler.vi"("error in (no error)"=w662) -> ()  [unwired: 4 in, 5 out]
                          }
                          frame #1 {
                            n445 = shared-variable "我的电脑\\200滑移力曲线.lvlib\\备用_1"(u16 0 ("备用1")) -> ()  [unwired: 1 in, 1 out]
                            n446 = shared-variable "我的电脑\\200滑移力曲线.lvlib\\备用_3"(u16 0 ("备用1")) -> ()  [unwired: 1 in, 1 out]
                          }
                        }
                      }
                    }
                  }
                  frame 1000 {
                    n447 = stacked-sequence {
                      frame #0 {
                        w703 = u32 16777216
                        w704 = "" ("传感器码")
                        w706 = ""
                        w708 = cluster{u32, u32}[] [{11776947, 11776947}, {11776947, 11776947}, {11776947, 11776947}, {11776947, 11776947}] ("颜色[4]")
                        w707 = "" ("传感器码")
                        n448 = shared-variable "我的电脑\\200滑移力曲线.lvlib\\设备状态"(u16 0 ("设备状态")) -> ()  [unwired: 1 in, 1 out]
                        n449 = Wait (ms)(milliseconds to wait=u32 300 ("等待时间（毫秒）")) -> ()  [unwired: 1 out]
                        n450 = shared-variable "我的电脑\\Global.lvlib\\传感器码"(w707) -> ()  [unwired: 1 in, 1 out]
                        n451 = local write "产品条码"(w707) -> ()
                        n452 = local write "产品条码 2"(w707) -> ()
                        n453 = local write "产品条码 3"(w707) -> ()
                        n454 = local write "产品条码 4"(w707) -> ()
                        n455 = local write "传感器上序状态"(w706) -> ()
                        n456 = local write "上柱管上序状态"(w706) -> ()
                        n457 = local write "传感器上序状态 3"(w706) -> ()
                        n458 = local write "上柱管上序状态 3"(w706) -> ()
                        n459 = property on="上柱管上序状态 2" class="Bool (严格)"("Colors [4]"=w708) -> ()  [unwired: 2 in, 2 out]
                        n460 = property on="传感器上序状态 2" class="Bool (严格)"("Colors [4]"=w708) -> ()  [unwired: 2 in, 2 out]
                        n461 = property on="传感器上序状态" class="Bool (严格)"("Colors [4]"=w708) -> ()  [unwired: 2 in, 2 out]
                        n462 = property on="上柱管上序状态" class="Bool (严格)"("Colors [4]"=w708) -> ()  [unwired: 2 in, 2 out]
                        n463 = local write "传感器码"(w704) -> ()
                        n464 = local write "管柱码状态"(w704) -> ()
                        n465 = local write "管柱二维码"(w704) -> ()
                        n466 = local write "传感器码状态"(w704) -> ()
                        n467 = property on="传感器码状态" class="Str"("Text.BGColor"=w703) -> ()  [unwired: 2 in, 2 out]
                        n468 = property on="管柱码状态" class="Str"("Text.BGColor"=w703) -> ()  [unwired: 2 in, 2 out]
                      }
                      frame #1 {
                        w712 = "请扫传感器码！" ("通知内容")
                        n469 = shared-variable "我的电脑\\200滑移力曲线.lvlib\\备用_1"(u16 1001 ("备用1")) -> ()  [unwired: 1 in, 1 out]
                        n470 = call "浮动通知.vi"("通知内容"=w712) -> ()  [unwired: 11 in]
                        n471 = call "输入框.vi"("提示信息"=w712) -> ("条形码输出"=w710:string)
                        "产品条码" <- w710
                        "产品条码 2" <- w710
                        "传感器码" <- w710
                        n472 = shared-variable "我的电脑\\Global.lvlib\\传感器码"(w710) -> ()  [unwired: 1 in, 1 out]
                      }
                    }
                  }
                  frame 1001 {
                    n473 = shared-variable "我的电脑\\Global.lvlib\\传感器码"() -> (w713:string)  [unwired: 1 in, 1 out]
                    n474 = String Length(string=w713) -> (length=w715:i32)
                    n475 = Greater?(x=w715, y=4) -> (0:w716:bool)
                    n476 = case shown="真" w716 {
                      frame False {
                      }
                      frame True {
                        n477 = shared-variable "我的电脑\\200滑移力曲线.lvlib\\备用_1"(u16 1100 ("备用1")) -> ()  [unwired: 1 in, 1 out]
                      }
                    }
                  }
                  frame 1100 {
                    n478 = global read "Global1.vi" "联机模式"() -> (w718:enum16{"单机", "追溯"})
                    n479 = case shown="\"追溯\"" w718 {
                      frame "单机", Default {
                        n480 = shared-variable "我的电脑\\200滑移力曲线.lvlib\\备用_1"(u16 1002 ("备用1")) -> ()  [unwired: 1 in, 1 out]
                      }
                      frame "追溯" {
                        n481 = stacked-sequence {
                          frame #0 {
                            n482 = shared-variable "我的电脑\\Global.lvlib\\传感器码"() -> (w725:string)  [unwired: 1 in, 1 out]
                            n483 = local read "productid"() -> (w722:string)
                            n484 = global read "Global1.vi" "联机模式"() -> (w741:enum16{"单机", "追溯"})
                            n485 = call "GetSQLstring.vi"("联机模式"=w741) -> ("错误输出"=w739:errorcluster, "连接字符串"=w740:string)  [unwired: 9 in]
                            n486 = call-poly <vilib>:"DB Tools Open Connection.vi"("error in (no error)"=w739, "connection information"=w740) -> ("error out"=w732:errorcluster, "connection reference"=w733:T6)  [unwired: 6 in]
                            n487 = Concatenate Strings("SELECT CODE_ID  FROM CODE  WHERE CODE_SENSOR ='" ("字符串"), w725, "'" ("字符串"), " AND PRODUCT_ID='" ("字符串"), w722, "'" ("字符串")) -> (w738:string)
                            "连接的字符串" <- w738
                            n488 = call-poly <vilib>:"DB Tools Execute Query.vi"("error in (no error)"=w732, "SQL query"=w738, "connection reference"=w733) -> ("error out"=w736:errorcluster, "recordset reference"=w737:T12)  [unwired: 5 in]
                            n489 = call-poly <vilib>:"DB Tools Fetch Recordset Data.vi"("error in (no error)"=w736, "recordset reference"=w737) -> ("error out"=w731:errorcluster, "recordset data"=w735:variant[][])  [unwired: 3 in, 1 out]
                            n490 = Variant To Data ("变体至数据转换")(error in=w731, type=string[][] [], Variant=w735) -> (data=w730:string[][])  [unwired: 1 out]
                            n491 = Index Array(array=w730, index (row)=0 ("索引 (行)")) -> (element=w728:string[])  [unwired: 1 in]
                            n492 = Index Array(array=w728, index=0 ("索引 (行)")) -> (element=w720:string)
                            n493 = local write "CODE_ID"(w720) -> ()
                          }
                          frame #1 {
                            w743 = "'" ("字符串")
                            n494 = local read "Fproductid_SENSOR"() -> (w748:string)
                            n495 = local read "Fproductid_MAIN"() -> (w746:string)
                            n496 = local read "CODE_ID"() -> (w744:string)
                            n497 = global read "Global1.vi" "联机模式"() -> (w764:enum16{"单机", "追溯"})
                            n498 = call "GetSQLstring.vi"("联机模式"=w764) -> ("错误输出"=w762:errorcluster, "连接字符串"=w763:string)  [unwired: 9 in]
                            n499 = call-poly <vilib>:"DB Tools Open Connection.vi"("error in (no error)"=w762, "connection information"=w763) -> ("error out"=w755:errorcluster, "connection reference"=w756:T6)  [unwired: 6 in]
                            n500 = Concatenate Strings("SELECT RESULT_VALUE FROM RESULT  WHERE (DEVICE_ID ='" ("字符串"), w748, "'  OR   DEVICE_ID ='" ("字符串"), w746, w743, " ) AND CODE_ID ='" ("字符串"), w744, w743) -> (w761:string)
                            "连接的字符串 2" <- w761
                            n501 = call-poly <vilib>:"DB Tools Execute Query.vi"("error in (no error)"=w755, "SQL query"=w761, "connection reference"=w756) -> ("error out"=w759:errorcluster, "recordset reference"=w760:T12)  [unwired: 5 in]
                            n502 = call-poly <vilib>:"DB Tools Fetch Recordset Data.vi"("error in (no error)"=w759, "recordset reference"=w760) -> ("error out"=w754:errorcluster, "recordset data"=w758:variant[][])  [unwired: 3 in, 1 out]
                            n503 = Variant To Data(error in=w754, type=string[][] [], Variant=w758) -> (data=w751:string[][])  [unwired: 1 out]
                            "传感器码" <- w751
                            n504 = Index Array(array=w751, index (row)=0 ("禁用的索引 (列)")) -> (element=w752:string[])  [unwired: 1 in]
                            n505 = Index Array(array=w752, index=0 ("索引 (行)")) -> (element=w750:string)
                            n506 = case shown="\"OK\"" w750 {
                              frame "假", Default {
                              }
                              frame "" {
                                w766 = "漏序" ("传感器上序状态")
                                w767 = cluster{u32, u32}[] [{16767232, 16767232}, {16767232, 16767232}, {16767232, 16767232}, {16767232, 16767232}] ("颜色[4]")
                                n507 = shared-variable "我的电脑\\200滑移力曲线.lvlib\\备用_1"(u16 5000 ("备用1")) -> ()  [unwired: 1 in, 1 out]
                                n508 = local write "传感器上序状态"(w766) -> ()
                                n509 = local write "传感器上序状态 3"(w766) -> ()
                                n510 = property on="传感器上序状态 2" class="Bool (严格)"("Colors [4]"=w767) -> ()  [unwired: 2 in, 2 out]
                                n511 = property on="传感器上序状态" class="Bool (严格)"("Colors [4]"=w767) -> ()  [unwired: 2 in, 2 out]
                                n512 = local write "传感器码状态"(w766) -> ()
                                n513 = property on="传感器码状态" class="Str"("Text.BGColor"=u32 16767232) -> ()  [unwired: 2 in, 2 out]
                              }
                              frame "OK" {
                                w770 = "合格" ("传感器上序状态")
                                w771 = cluster{u32, u32}[] [{6618880, 6618880}, {6618880, 6618880}, {6618880, 6618880}, {6618880, 6618880}] ("颜色[4]")
                                n514 = shared-variable "我的电脑\\200滑移力曲线.lvlib\\备用_1"(u16 1002 ("备用1")) -> ()  [unwired: 1 in, 1 out]
                                n515 = local write "传感器上序状态"(w770) -> ()
                                n516 = local write "传感器上序状态 3"(w770) -> ()
                                n517 = property on="传感器上序状态 2" class="Bool (严格)"("Colors [4]"=w771) -> ()  [unwired: 2 in, 2 out]
                                n518 = property on="传感器上序状态" class="Bool (严格)"("Colors [4]"=w771) -> ()  [unwired: 2 in, 2 out]
                                n519 = property on="传感器码状态" class="Str"("Text.BGColor"=u32 6618880) -> ()  [unwired: 2 in, 2 out]
                                n520 = local write "传感器码状态"(w770) -> ()
                              }
                              frame "NG" {
                                w773 = "不合格" ("传感器上序状态")
                                w775 = cluster{u32, u32}[] [{16711680, 16711680}, {16711680, 16711680}, {16711680, 16711680}, {16711680, 16711680}] ("颜色[4]")
                                n521 = shared-variable "我的电脑\\200滑移力曲线.lvlib\\备用_1"(u16 5000 ("备用1")) -> ()  [unwired: 1 in, 1 out]
                                n522 = local write "传感器上序状态"(w773) -> ()
                                n523 = local write "传感器上序状态 3"(w773) -> ()
                                n524 = property on="传感器上序状态 2" class="Bool (严格)"("Colors [4]"=w775) -> ()  [unwired: 2 in, 2 out]
                                n525 = property on="传感器上序状态" class="Bool (严格)"("Colors [4]"=w775) -> ()  [unwired: 2 in, 2 out]
                                n526 = local write "传感器码状态"(w773) -> ()
                                n527 = property on="传感器码状态" class="Str"("Text.BGColor"=u32 16711680) -> ()  [unwired: 2 in, 2 out]
                              }
                            }
                          }
                        }
                      }
                    }
                  }
                  frame 1002 {
                    n528 = stacked-sequence {
                      frame #0 {
                        n529 = Wait (ms)(milliseconds to wait=u32 300 ("等待时间（毫秒）")) -> ()  [unwired: 1 out]
                        n530 = shared-variable "我的电脑\\Global.lvlib\\工位追溯码"("" ("传感器码")) -> ()  [unwired: 1 in, 1 out]
                      }
                      frame #1 {
                        w781 = "请扫上柱管码！" ("通知内容")
                        n531 = shared-variable "我的电脑\\200滑移力曲线.lvlib\\备用_1"(u16 1003 ("备用1")) -> ()  [unwired: 1 in, 1 out]
                        n532 = call "浮动通知.vi"("通知内容"=w781) -> ()  [unwired: 11 in]
                        n533 = call "输入框.vi"("提示信息"=w781) -> ("条形码输出"=w779:string)
                        "产品条码 4" <- w779
                        "产品条码 3" <- w779
                        "管柱二维码" <- w779
                        n534 = shared-variable "我的电脑\\Global.lvlib\\工位追溯码"(w779) -> ()  [unwired: 1 in, 1 out]
                      }
                      frame #2 {
                        n535 = vi-ref "滑移力曲线.vi"() -> (w783:refnum<vi>)
                        n536 = call "CallVI.vi"("VI引用"=w783, "状态"=T2."Hidden") -> ()  [unwired: 12 in, 2 out]
                      }
                      frame #3 {
                        n537 = for {
                          N: 2 -> [_]
                          tunnel: [cluster{dbl[], dbl[]} {[], []}] -> w786 mode=indexing
                        }
                        n538 = local read "滑移力复检曲线"() -> (w785:cluster{dbl[], dbl[]}[])
                        n539 = Replace Array Subset(array=w785, new element=w786) -> (w787:cluster{dbl[], dbl[]}[])  [unwired: 1 in]
                        n540 = local write "滑移力复检曲线"(w787) -> ()
                      }
                      frame #4 {
                        w791 = -2
                        n541 = control-ref of="表格控件"() -> (w792:refnum<vi>)
                        n542 = Bundle(w791, w791) -> (w793:cluster{i32, i32})  [unwired: 1 in]
                        n543 = property class="Tbl (严格)"(reference=w792, "Row Headers[]"=string[] [] ("行首字符串[]")) -> ()  [unwired: 1 in, 2 out]
                        n544 = property class="Tbl (严格)"(reference=w792, "Active Cell"=w793, "Cell BG Color"=u32 16777216 ("活动单元格:单元格背景色")) -> ()  [unwired: 1 in, 2 out]
                        "表格控件" <- string[][] [] ("判定")
                      }
                    }
                  }
                  frame 1003 {
                    n545 = shared-variable "我的电脑\\Global.lvlib\\工位追溯码"() -> (w795:string)  [unwired: 1 in, 1 out]
                    n546 = String Length(string=w795) -> (length=w797:i32)
                    n547 = Greater?(x=w797, y=4) -> (0:w798:bool)
                    n548 = case shown="真" w798 {
                      frame False {
                      }
                      frame True {
                        n549 = shared-variable "我的电脑\\200滑移力曲线.lvlib\\备用_1"(u16 1200 ("备用1")) -> ()  [unwired: 1 in, 1 out]
                      }
                    }
                  }
                  frame 1200 {
                    n550 = global read "Global1.vi" "联机模式"() -> (w800:enum16{"单机", "追溯"})
                    n551 = case shown="\"追溯\"" w800 {
                      frame "单机", Default {
                        n552 = shared-variable "我的电脑\\200滑移力曲线.lvlib\\备用_1"(u16 1004 ("备用1")) -> ()  [unwired: 1 in, 1 out]
                      }
                      frame "追溯" {
                        n553 = stacked-sequence {
                          frame #0 {
                            n554 = shared-variable "我的电脑\\Global.lvlib\\工位追溯码"() -> (w802:string)  [unwired: 1 in, 1 out]
                            n555 = local read "productid"() -> (w805:string)
                            n556 = global read "Global1.vi" "联机模式"() -> (w823:enum16{"单机", "追溯"})
                            n557 = call "GetSQLstring.vi"("联机模式"=w823) -> ("错误输出"=w821:errorcluster, "连接字符串"=w822:string)  [unwired: 9 in]
                            n558 = call-poly <vilib>:"DB Tools Open Connection.vi"("error in (no error)"=w821, "connection information"=w822) -> ("error out"=w814:errorcluster, "connection reference"=w815:T6)  [unwired: 6 in]
                            n559 = Concatenate Strings("SELECT CODE_ID  FROM CODE  WHERE CODE_MAIN ='", w802, "'" ("字符串"), " AND PRODUCT_ID='" ("字符串"), w805, "'" ("字符串")) -> (w820:string)
                            n560 = call-poly <vilib>:"DB Tools Execute Query.vi"("error in (no error)"=w814, "SQL query"=w820, "connection reference"=w815) -> ("error out"=w818:errorcluster, "recordset reference"=w819:T12)  [unwired: 5 in]
                            n561 = call-poly <vilib>:"DB Tools Fetch Recordset Data.vi"("error in (no error)"=w818, "recordset reference"=w819) -> ("error out"=w813:errorcluster, "recordset data"=w817:variant[][])  [unwired: 3 in, 1 out]
                            n562 = Variant To Data(error in=w813, type=string[][] [], Variant=w817) -> (data=w812:string[][])  [unwired: 1 out]
                            n563 = Index Array(array=w812, index (row)=0 ("索引 (行)")) -> (element=w810:string[])  [unwired: 1 in]
                            n564 = Index Array(array=w810, index=0 ("索引 (行)")) -> (element=w808:string)
                            n565 = local write "CODE_ID 2"(w808) -> ()
                          }
                          frame #1 {
                            w825 = "'" ("字符串")
                            n566 = local read "Fproductid_MAIN"() -> (w831:string)
                            n567 = local read "CODE_ID 2"() -> (w826:string)
                            n568 = local read "Fproductid_SENSOR"() -> (w828:string)
                            n569 = global read "Global1.vi" "联机模式"() -> (w846:enum16{"单机", "追溯"})
                            n570 = call "GetSQLstring.vi"("联机模式"=w846) -> ("错误输出"=w844:errorcluster, "连接字符串"=w845:string)  [unwired: 9 in]
                            n571 = call-poly <vilib>:"DB Tools Open Connection.vi"("error in (no error)"=w844, "connection information"=w845) -> ("error out"=w837:errorcluster, "connection reference"=w838:T6)  [unwired: 6 in]
                            n572 = Concatenate Strings("SELECT RESULT_VALUE FROM RESULT  WHERE (DEVICE_ID ='", w831, w825, " OR  DEVICE_ID='", w828, w825, ")  AND CODE_ID ='" ("字符串"), w826, w825) -> (w843:string)
                            n573 = call-poly <vilib>:"DB Tools Execute Query.vi"("error in (no error)"=w837, "SQL query"=w843, "connection reference"=w838) -> ("error out"=w841:errorcluster, "recordset reference"=w842:T12)  [unwired: 5 in]
                            n574 = call-poly <vilib>:"DB Tools Fetch Recordset Data.vi"("error in (no error)"=w841, "recordset reference"=w842) -> ("error out"=w836:errorcluster, "recordset data"=w840:variant[][])  [unwired: 3 in, 1 out]
                            n575 = Variant To Data(error in=w836, type=string[][] [], Variant=w840) -> (data=w833:string[][])  [unwired: 1 out]
                            "二维码" <- w833
                            n576 = Index Array(array=w833, index (row)=0 ("索引 (行)")) -> (element=w834:string[])  [unwired: 1 in]
                            n577 = Index Array(array=w834, index=0 ("索引 (行)")) -> (element=w832:string)
                            n578 = case shown="\"NG\"" w832 {
                              frame "假", Default {
                              }
                              frame "" {
                                w848 = "漏序" ("上柱管上序状态")
                                w850 = cluster{u32, u32}[] [{16767232, 16767232}, {16767232, 16767232}, {16767232, 16767232}, {16767232, 16767232}] ("颜色[4]")
                                n579 = shared-variable "我的电脑\\200滑移力曲线.lvlib\\备用_1"(u16 5001 ("备用1")) -> ()  [unwired: 1 in, 1 out]
                                n580 = local write "上柱管上序状态"(w848) -> ()
                                n581 = local write "上柱管上序状态 3"(w848) -> ()
                                n582 = property on="上柱管上序状态 2" class="Bool (严格)"("Colors [4]"=w850) -> ()  [unwired: 2 in, 2 out]
                                n583 = property on="上柱管上序状态" class="Bool (严格)"("Colors [4]"=w850) -> ()  [unwired: 2 in, 2 out]
                                n584 = property on="管柱码状态" class="Str"("Text.BGColor"=u32 16767232) -> ()  [unwired: 2 in, 2 out]
                                n585 = local write "管柱码状态"(w848) -> ()
                              }
                              frame "OK" {
                                w851 = "合格" ("上柱管上序状态")
                                w853 = cluster{u32, u32}[] [{6618880, 6618880}, {6618880, 6618880}, {6618880, 6618880}, {6618880, 6618880}] ("颜色[4]")
                                n586 = shared-variable "我的电脑\\200滑移力曲线.lvlib\\备用_1"(u16 1004 ("备用1")) -> ()  [unwired: 1 in, 1 out]
                                n587 = local write "上柱管上序状态"(w851) -> ()
                                n588 = local write "上柱管上序状态 3"(w851) -> ()
                                n589 = property on="上柱管上序状态 2" class="Bool (严格)"("Colors [4]"=w853) -> ()  [unwired: 2 in, 2 out]
                                n590 = property on="上柱管上序状态" class="Bool (严格)"("Colors [4]"=w853) -> ()  [unwired: 2 in, 2 out]
                                n591 = property on="管柱码状态" class="Str"("Text.BGColor"=u32 6618880) -> ()  [unwired: 2 in, 2 out]
                                n592 = local write "管柱码状态"(w851) -> ()
                              }
                              frame "NG" {
                                w856 = "不合格" ("上柱管上序状态")
                                w857 = cluster{u32, u32}[] [{16711680, 16711680}, {16711680, 16711680}, {16711680, 16711680}, {16711680, 16711680}] ("颜色[4]")
                                n593 = shared-variable "我的电脑\\200滑移力曲线.lvlib\\备用_1"(u16 5001 ("备用1")) -> ()  [unwired: 1 in, 1 out]
                                n594 = local write "上柱管上序状态"(w856) -> ()
                                n595 = local write "上柱管上序状态 3"(w856) -> ()
                                n596 = property on="上柱管上序状态 2" class="Bool (严格)"("Colors [4]"=w857) -> ()  [unwired: 2 in, 2 out]
                                n597 = property on="上柱管上序状态" class="Bool (严格)"("Colors [4]"=w857) -> ()  [unwired: 2 in, 2 out]
                                n598 = local write "管柱码状态"(w856) -> ()
                                n599 = property on="管柱码状态" class="Str"("Text.BGColor"=u32 16711680) -> ()  [unwired: 2 in, 2 out]
                              }
                            }
                          }
                        }
                      }
                    }
                  }
                }
              }
            }
            n600 = Format Date/Time String(time format string (%c)="%H:%M:%S" ("时间格式字符串(%c)")) -> (date/time string=→"时间":string)  [unwired: 2 in]
          }
          event "删除": Value Change {
            n601 = event-data() -> ("NewVal"=w860:bool)  [unwired: 1 in, 5 out]
            n602 = case shown="真" w860 {
              tunnel: w859 -> [_ w862]
              frame False {
              }
              frame True {
                n603 = Concatenate Strings("确认删除“", "请选择要删除的产品", "”吗？") -> (w864:string)
                n604 = Two Button Dialog(message=w864) -> (T button?=w863:bool)  [unwired: 2 in]
                n605 = case shown="真" w863 {
                  tunnel: w862 -> [_ w868]
                  tunnel: "请选择要删除的产品" -> [_ w867]
                  frame False {
                  }
                  frame True {
                    n606 = call <vilib>:"Open Config Data.vi"("configuration file path"=w868) -> ("error out"=w870:errorcluster, "refnum"=w873:T5)  [unwired: 8 in, 1 out]
                    n607 = call <vilib>:"Remove Section.vi"("section"=w867, "error in (no error)"=w870, "refnum"=w873) -> ("error out"=w872:errorcluster, "section exists?"=w869:bool, "refnum out"=w871:T5)  [unwired: 6 in]
                    n608 = call <vilib>:"Close Config Data.vi"("error in (no error)"=w872, "refnum"=w871) -> ()  [unwired: 8 in, 2 out]
                    n609 = case shown="真" w869 {
                      frame False {
                        n610 = One Button Dialog(message="删除失败！\n请确认产品存在！" ("消息")) -> ()  [unwired: 1 in, 1 out]
                      }
                      frame True {
                        n611 = One Button Dialog(message="删除成功！" ("消息")) -> ()  [unwired: 1 in, 1 out]
                      }
                    }
                  }
                }
              }
            }
          }
          event "确定": Value Change {
            n612 = event-data() -> ("NewVal"=w876:bool)  [unwired: 1 in, 5 out]
            n613 = case shown="真" w876 {
              frame False {
              }
              frame True {
                n614 = stacked-sequence {
                  seq-local: [w880 _ _ _ _ _] -> [_ _ _ _ _ _]
                  frame #0 {
                    n615 = shared-variable "我的电脑\\200滑移力曲线.lvlib\\备用_3"(u16 0 ("备用1")) -> ()  [unwired: 1 in, 1 out]
                    n616 = global read "Global1.vi" "联机模式"() -> (w877:enum16{"单机", "追溯"})
                    n617 = case shown="\"追溯\"" w877 {
                      frame "单机", Default {
                      }
                      frame "追溯" {
                        n618 = local read "产品型号"() -> (w889:string)
                        n619 = call "Get_Device_ID.vi"() -> ("Device_ID"=→"deviceid":string)  [unwired: 10 in, 1 out]
                        n620 = call "GET_PRODUCT_ID.vi"("PRODFUCT_NAME"=w889) -> ("PRODUCT_ID"=w888:string)  [unwired: 10 in]
                        "productid" <- w888
                        n621 = call "查询前序设备.vi"("PRODUCT_ID"=w888) -> ("前序工位"=w887:string[])  [unwired: 10 in]
                        "前序工位" <- w887
                        n622 = Index Array(array=w887, index #1=0 ("索引"), index #2=1 ("索引")) -> (element #1=→"Fproductid_SENSOR":string, element #2=→"Fproductid_MAIN":string)
                      }
                    }
                    n623 = local read "产品型号"() -> (w879:string)
                    "产品型号" <- w879
                    n624 = shared-variable "我的电脑\\Global.lvlib\\产品型号"(w879) -> ()  [unwired: 1 in, 1 out]
                    n625 = String Subset(string=w879, offset (0)=u16 2 ("偏移量(0)"), length (rest)=u16 4 ("长度（剩余）")) -> (substring=w880:string)
                    n626 = Decimal String To Number(string=w880) -> ()  [unwired: 2 in, 2 out]
                  }
                  frame #1 {
                    n627 = global read "Global1.vi" "联机模式"() -> (w898:enum16{"单机", "追溯"})
                    n628 = local read "用户名"() -> (w891:string)
                    n629 = call "GetSQLstring.vi"("联机模式"=w898) -> ("错误输出"=w900:errorcluster, "连接字符串"=w899:string)  [unwired: 9 in]
                    n630 = call-poly <vilib>:"DB Tools Open Connection.vi"("error in (no error)"=w900, "connection information"=w899) -> ("error out"=w906:errorcluster, "connection reference"=w905:T6)  [unwired: 6 in]
                    n631 = Concatenate Strings("SELECT USER_ID FROM [User]  WHERE USER_NAME ='", w891, "'" ("字符串")) -> (w901:string)
                    n632 = call-poly <vilib>:"DB Tools Execute Query.vi"("error in (no error)"=w906, "SQL query"=w901, "connection reference"=w905) -> ("error out"=w903:errorcluster, "recordset reference"=w902:T12)  [unwired: 5 in]
                    n633 = call-poly <vilib>:"DB Tools Fetch Recordset Data.vi"("error in (no error)"=w903, "recordset reference"=w902) -> ("error out"=w907:errorcluster, "recordset data"=w904:variant[][])  [unwired: 3 in, 1 out]
                    n634 = Variant To Data(error in=w907, type=string[][] [], Variant=w904) -> (data=w908:string[][])  [unwired: 1 out]
                    n635 = Index Array(array=w908, index (row)=0 ("索引 (行)")) -> (element=w909:string[])  [unwired: 1 in]
                    n636 = Index Array(array=w909, index=0 ("索引 (行)")) -> (element=→"USER_ID":string)
                  }
                  frame #2 {
                    n637 = Index Array(array="坐标参数", index (row) #1=0 ("索引 (行)"), index (row) #2=1 ("索引 (行)")) -> (element #1=w929:string[], element #2=w928:string[])  [unwired: 2 in]
                    n638 = Index Array(array=w929, index=1 ("索引 (行)")) -> (element=w927:string)
                    n639 = Index Array(array=w929, index=2 ("索引 (行)")) -> (element=w926:string)
                    n640 = Index Array(array=w928, index=1 ("索引 (行)")) -> (element=w925:string)
                    n641 = Index Array(array=w928, index=2 ("索引 (行)")) -> (element=w924:string)
                    n642 = Fract/Exp String To Number(string=w927) -> (number=w923:dbl)  [unwired: 3 in, 1 out]
                    n643 = Fract/Exp String To Number(string=w926) -> (number=w922:dbl)  [unwired: 3 in, 1 out]
                    n644 = Fract/Exp String To Number(string=w925) -> (number=w920:dbl)  [unwired: 3 in, 1 out]
                    n645 = Fract/Exp String To Number(string=w924) -> (number=w921:dbl)  [unwired: 3 in, 1 out]
                    n646 = property on="滑移力复检曲线" class="XYGraph (严格)"("XScale.Minimum"=w923) -> ()  [unwired: 2 in, 2 out]
                    n647 = property on="滑移力复检曲线" class="XYGraph (严格)"("XScale.Maximum"=w922) -> ()  [unwired: 2 in, 2 out]
                    n648 = property on="滑移力复检曲线" class="XYGraph (严格)"("YScale.Minimum"=w920) -> ()  [unwired: 2 in, 2 out]
                    n649 = property on="滑移力复检曲线" class="XYGraph (严格)"("YScale.Maximum"=w921) -> ()  [unwired: 2 in, 2 out]
                    n650 = local read "判定项"() -> (w912:string[][])
                    n651 = local read "滑移力判定项 2"() -> (w919:string[][])
                    n652 = for {
                      tunnel: w912 -> [w943] mode=indexing
                      tunnel: [w937] -> w911 mode=indexing
                      n653 = Index Array(array=w943) -> (element #1=w940:string, element #2=w942:string, element #3=w941:string)  [unwired: 3 in]
                      n654 = Fract/Exp String To Number(string=w942) -> (number=w939:dbl)  [unwired: 3 in, 1 out]
                      n655 = Fract/Exp String To Number(string=w941) -> (number=w938:dbl)  [unwired: 3 in, 1 out]
                      n656 = Bundle(w940, w939, w938) -> (w937:cluster{string, dbl, dbl})  [unwired: 1 in]
                    }
                    n657 = Index Array(array=w919) -> (element #1=w918:string[], element #2=w915:string[])  [unwired: 4 in]
                    n658 = Array To Cluster(array=w911) -> (cluster=w910:T13)
                    n659 = Index Array(array=w918) -> (element=w917:string)  [unwired: 1 in]
                    n660 = global write "Global.vi" "判定参数"(w910) -> ()
                    n661 = Index Array(array=w915) -> (element=w914:string)  [unwired: 1 in]
                    n662 = Fract/Exp String To Number(string=w917) -> (number=w916:dbl)  [unwired: 3 in, 1 out]
                    n663 = Fract/Exp String To Number(string=w914) -> (number=w913:dbl)  [unwired: 3 in, 1 out]
                    n664 = global write "A131258.vi" "拉力"(w916) -> ()
                    n665 = global write "A131258.vi" "压力"(w913) -> ()
                  }
                  frame #3 {
                    n666 = local read "判定项"() -> (w966:string[][])
                    n667 = Index Array(array=w966, index (row) #1=0 ("索引 (行)"), index (row) #2=0 ("索引 (行)"), index (row) #3=1 ("索引 (行)"), index (row) #4=1 ("索引 (行)")) -> (element #1=w965:string[], element #2=w964:string[], element #3=w963:string[], element #4=w962:string[])  [unwired: 4 in]
                    n668 = Index Array(array=w965, index=1 ("索引")) -> (element=w961:string)
                    n669 = Index Array(array=w964, index=2 ("索引")) -> (element=w960:string)
                    n670 = Index Array(array=w963, index=1 ("索引")) -> (element=w959:string)
                    n671 = Index Array(array=w962, index=2 ("索引")) -> (element=w958:string)
                    n672 = local read "滑移力复检曲线"() -> (w944:cluster{dbl[], dbl[]}[])
                    n673 = Fract/Exp String To Number(string=w961) -> (number=w949:dbl)  [unwired: 3 in, 1 out]
                    n674 = Fract/Exp String To Number(string=w960) -> (number=w948:dbl)  [unwired: 3 in, 1 out]
                    n675 = Fract/Exp String To Number(string=w959) -> (number=w947:dbl)  [unwired: 3 in, 1 out]
                    n676 = Fract/Exp String To Number(string=w958) -> (number=w946:dbl)  [unwired: 3 in, 1 out]
                    n677 = for {
                      tunnel: w949 -> [w972]
                      tunnel: w948 -> [w971]
                      tunnel: w947 -> [w970]
                      tunnel: w946 -> [w969]
                      tunnel: [w968] -> w945 mode=indexing
                      tunnel: w944 -> [w967] mode=indexing
                      i -> [w973]
                      n678 = case shown="2" w973 {
                        tunnel: w972 -> [_ w981]
                        tunnel: w971 -> [_ w980]
                        tunnel: w970 -> [_ w975]
                        tunnel: w969 -> [_ w976]
                        tunnel: [w974 w977] -> w968
                        tunnel: w967 -> [w974 _]
                        frame Default {
                        }
                        frame 2 {
                          n679 = Build Array(w981, w981, w980, w980, w981) -> (w979:dbl[])
                          n680 = Build Array(w976, w975, w975, w976, w976) -> (w978:dbl[])
                          n681 = Bundle(w979, w978) -> (w977:cluster{dbl[], dbl[]})  [unwired: 1 in]
                        }
                      }
                    }
                    n682 = local write "滑移力复检曲线"(w945) -> ()
                  }
                  frame #4 {
                    n683 = local read "判定项"() -> (w982:string[][])
                    n684 = Index Array(array=w982, index (row) #1=4 ("索引 (行)"), index (row) #2=4 ("索引 (行)"), index (row) #3=5 ("索引 (行)"), index (row) #4=5 ("索引 (行)")) -> (element #1=w1002:string[], element #2=w1001:string[], element #3=w1000:string[], element #4=w999:string[])  [unwired: 4 in]
                    n685 = Index Array(array=w1002, index=1 ("索引")) -> (element=w994:string)
                    n686 = Index Array(array=w1001, index=2 ("索引")) -> (element=w993:string)
                    n687 = Index Array(array=w1000, index=1 ("索引")) -> (element=w992:string)
                    n688 = Index Array(array=w999, index=2 ("索引")) -> (element=w991:string)
                    n689 = local read "滑移力复检曲线"() -> (w1004:cluster{dbl[], dbl[]}[])
                    n690 = Fract/Exp String To Number(string=w994) -> (number=w998:dbl)  [unwired: 3 in, 1 out]
                    n691 = Fract/Exp String To Number(string=w993) -> (number=w997:dbl)  [unwired: 3 in, 1 out]
                    n692 = Fract/Exp String To Number(string=w992) -> (number=w995:dbl)  [unwired: 3 in, 1 out]
                    n693 = Fract/Exp String To Number(string=w991) -> (number=w996:dbl)  [unwired: 3 in, 1 out]
                    n694 = for {
                      tunnel: w995 -> [w1011]
                      tunnel: w996 -> [w1010]
                      tunnel: w997 -> [w1009]
                      tunnel: w998 -> [w1008]
                      tunnel: [w1007] -> w1003 mode=indexing
                      tunnel: w1004 -> [w1005] mode=indexing
                      i -> [w1006]
                      n695 = case shown="3" w1006 {
                        tunnel: w1011 -> [_ w1019]
                        tunnel: w1010 -> [_ w1018]
                        tunnel: w1009 -> [_ w1017]
                        tunnel: w1008 -> [_ w1016]
                        tunnel: [w1012 w1013] -> w1007
                        tunnel: w1005 -> [w1012 _]
                        frame Default {
                        }
                        frame 3 {
                          n696 = Build Array(w1016, w1016, w1017, w1017, w1016) -> (w1015:dbl[])
                          n697 = Build Array(w1019, w1018, w1018, w1019, w1019) -> (w1014:dbl[])
                          n698 = Bundle(w1015, w1014) -> (w1013:cluster{dbl[], dbl[]})  [unwired: 1 in]
                        }
                      }
                    }
                    n699 = local write "滑移力复检曲线"(w1003) -> ()
                  }
                  frame #5 {
                    n700 = stacked-sequence {
                      frame #0 {
                        w1020 = "参数装载成功！" ("消息")
                        n701 = call "浮动通知.vi"("通知内容"=w1020) -> ()  [unwired: 11 in]
                        n702 = One Button Dialog(message=w1020) -> ()  [unwired: 1 in, 1 out]
                      }
                      frame #1 {
                        n703 = local write "选项卡控件 2"(enum32{"管柱总成装配", "管柱总成装配右", "滑移力曲线", "参数查看"}."滑移力曲线" ("选项卡控件 2")) -> ()
                      }
                    }
                  }
                }
              }
            }
          }
          event "添加": Value Change {
            n704 = event-data() -> ("NewVal"=w1026:bool)  [unwired: 1 in]
            n705 = local read "请输入添加的产品名称"() -> (w1024:string)
            n706 = call <vilib>:"Trim Whitespace.vi"("string"=w1024) -> ("trimmed string"=w1022:string)  [unwired: 1 in]
            n707 = case shown="默认" w1022 {
              tunnel: w1025 -> [w1029 _]
              tunnel: w1026 -> [w1028 _]
              tunnel: w1023 -> [w1027 _]
              frame Default {
                n708 = case shown="真" w1028 {
                  tunnel: w1029 -> [_ w1031]
                  tunnel: w1027 -> [_ w1030]
                  frame False {
                  }
                  frame True {
                    n709 = for {
                      tunnel: w1031 -> [w1036]
                      tunnel: w1030 -> [w1033] mode=indexing
                      n710 = call "Read_Write ParaINI File.vi"("Mode"=enum16{"Read", "Write"}."Write", "Section"="请输入添加的产品名称", "Filepath"=w1036, "Ctl Refnum"=w1033) -> ("error out"=w1032:errorcluster)  [unwired: 7 in]
                      n711 = case shown="错误 .." w1032 {
                        frame No Error {
                          n712 = One Button Dialog(message="添加成功！" ("消息")) -> ()  [unwired: 1 in, 1 out]
                        }
                        frame Error {
                          n713 = One Button Dialog(message="添加失败！" ("消息")) -> ()  [unwired: 1 in, 1 out]
                        }
                      }
                    }
                  }
                }
              }
              frame "" {
                w1039 = 64 items=["None"=0, "Hand, Error, Stop"=16, "Question"=32, "Exclamation, Warning"=48, "Asterisk, Information"=64] ("icon")
                w1040 = 0 items=["OK", "OKCancel", "AbortRetryIgnore", "YesNoCancel", "YesNo", "RetryCancel"] ("buttons")
                n714 = call "信息框（标题、文本、图标）.vi"("icon"=w1039, "buttons"=w1040, "caption"="添加失败", "text"="请输入产品名称!") -> ()  [unwired: 6 in, 2 out]
              }
            }
          }
          event "产品型号", "请选择要删除的产品": Value Change {
            n715 = event-data() -> ()  [unwired: 1 in, 6 out]
            n716 = stacked-sequence {
              tunnel: w1044 -> [_ w1046]
              tunnel: w1043 -> [_ w1045]
              frame #0 {
              }
              frame #1 {
                n717 = for {
                  tunnel: w1046 -> [w1050]
                  tunnel: w1045 -> [w1047] mode=indexing
                  n718 = local read "产品型号"() -> (w1048:string)
                  n719 = call "Read_Write ParaINI File.vi"("Mode"=enum16{"Read", "Write"}."Read", "Section"=w1048, "Filepath"=w1050, "Ctl Refnum"=w1047) -> ()  [unwired: 7 in, 1 out]
                }
              }
            }
          }
          event "退出": Value Change {
            n720 = event-data() -> ()  [unwired: 1 in, 6 out]
            n721 = control-ref of="本VI"() -> (w1053:refnum<vi>)
            n722 = invoke class="VI" method="FP.Close"(reference=w1053) -> (reference out=w1051:refnum<vi>, error out=w1052:errorcluster)  [unwired: 2 in, 1 out]
            n723 = Close Reference(reference=w1051, error in (no error)=w1052) -> ()  [unwired: 1 out]
          }
          event "更新": Value Change {
            n724 = event-data() -> ("NewVal"=w1056:bool)  [unwired: 1 in]
            n725 = case shown="真" w1056 {
              tunnel: w1055 -> [_ w1059]
              tunnel: w1054 -> [_ w1057]
              frame False {
              }
              frame True {
                n726 = for {
                  tunnel: w1059 -> [w1064]
                  tunnel: [w1063] -> w1058
                  tunnel: w1057 -> [w1060] mode=indexing
                  n727 = local read "产品型号"() -> (w1061:string)
                  n728 = call "Read_Write ParaINI File.vi"("Mode"=enum16{"Read", "Write"}."Write", "Section"=w1061, "Filepath"=w1064, "Ctl Refnum"=w1060) -> ("error out"=w1063:errorcluster)  [unwired: 7 in]
                }
                n729 = case shown="无错误" w1058 {
                  frame No Error {
                    n730 = call "浮动通知.vi"("通知内容"="更新成功！") -> ()  [unwired: 11 in]
                  }
                  frame Error {
                    n731 = call "浮动通知.vi"("通知内容"="更新失败！") -> ()  [unwired: 11 in]
                  }
                }
              }
            }
          }
          event "请输入添加的产品名称": Value Change {
            n732 = event-data() -> ("NewVal"=w1068:string)  [unwired: 1 in, 5 out]
            n733 = control-ref of="产品型号"() -> (w1067:refnum<vi>)
            n734 = property on="属性节点" class="CmbBox"(reference=w1067) -> ("Strings[]"=w1069:string[])  [unwired: 1 in, 2 out]
            n735 = for {
              tunnel: w1068 -> [w1070]
              tunnel: w1069 -> [w1071] mode=indexing
              n736 = Equal?(x=w1070, y=w1071) -> (x = y?=w1072:bool)
              n737 = case shown="真" w1072 {
                tunnel: w1070 -> [_ w1073]
                frame False {
                }
                frame True {
                  n738 = stacked-sequence {
                    tunnel: w1073 -> [w1079 _]
                    frame #0 {
                      w1074 = 64 items=["None"=0, "Hand, Error, Stop"=16, "Question"=32, "Exclamation, Warning"=48, "Asterisk, Information"=64] ("icon")
                      w1075 = 0 items=["OK", "OKCancel", "AbortRetryIgnore", "YesNoCancel", "YesNo", "RetryCancel"] ("buttons")
                      n739 = Concatenate Strings("已经存在产品”" ("text"), w1079, "“\n请勿重复添加！" ("字符串")) -> (w1077:string)
                      n740 = call "信息框（标题、文本、图标）.vi"("icon"=w1074, "buttons"=w1075, "caption"="产品重复", "text"=w1077) -> ()  [unwired: 6 in, 2 out]
                    }
                    frame #1 {
                      n741 = local write "请输入添加的产品名称"("" ("请输入添加的产品名称")) -> ()
                    }
                  }
                }
              }
            }
          }
          event Panel Close? {
            n742 = event-data() -> ()  [unwired: 1 in, 4 out]
            n743 = control-ref of="本VI"() -> (w1087:refnum<vi>)
            n744 = vi-ref "client.vi"() -> (w1082:refnum<vi>)
            n745 = global write "Global.vi" "程序关闭"(TRUE ("程序关闭")) -> ()
            n746 = invoke class="VI" method="FP.Close"(reference=w1087) -> (reference out=w1085:refnum<vi>, error out=w1086:errorcluster)  [unwired: 2 in, 1 out]
            n747 = invoke class="VI" method="FP.Close"(reference=w1082) -> (reference out=w1083:refnum<vi>, error out=w1084:errorcluster)  [unwired: 2 in, 1 out]
            n748 = Close Reference(reference=w1085, error in (no error)=w1086) -> ()  [unwired: 1 out]
            n749 = Close Reference(reference=w1083, error in (no error)=w1084) -> ()  [unwired: 1 out]
            n750 = event-data("Discard?"=TRUE ("放弃？")) -> ()  [unwired: 1 in, 1 out]
          }
          event "进入用户管理": Value Change {
            n751 = event-data() -> ()  [unwired: 1 in, 6 out]
            n752 = vi-ref "User_manager.vi"() -> (w1091:refnum<vi>)
            n753 = call "CallVI.vi"("VI引用"=w1091, "状态"=T2."Maximized") -> ()  [unwired: 12 in, 2 out]
          }
          event "设备故障", "设备故障2": Value Change {
            n754 = event-data() -> ()  [unwired: 1 in, 6 out]
            n755 = call "状态改变.vi"("设备状态"=enum16{"设备离线", "设备正常", "设备缺料", "设备故障", "质量报警"}."设备故障") -> ()  [unwired: 11 in]
          }
          event "设备缺料", "设备缺料2": Value Change {
            n756 = event-data() -> ()  [unwired: 1 in, 6 out]
            n757 = call "状态改变.vi"("设备状态"=enum16{"设备离线", "设备正常", "设备缺料", "设备故障", "质量报警"}."设备缺料") -> ()  [unwired: 11 in]
          }
          event "质量报警", "质量报警2": Value Change {
            n758 = event-data() -> ()  [unwired: 1 in, 6 out]
            n759 = call "状态改变.vi"("设备状态"=enum16{"设备离线", "设备正常", "设备缺料", "设备故障", "质量报警"}."质量报警") -> ()  [unwired: 11 in]
          }
          event "产品型号": Mouse Enter {
            n760 = event-data() -> ()  [unwired: 1 in, 1 out]
            n761 = call <vilib>:"Open Config Data.vi"("configuration file path"=w1097) -> ("refnum"=w1096:T5)  [unwired: 8 in, 2 out]
            n762 = call <vilib>:"Get Section Names.vi"("refnum"=w1096) -> ("section names"=w1095:string[])  [unwired: 8 in, 2 out]
            n763 = property on="产品型号" class="CmbBox"("Strings[]"=w1095) -> ()  [unwired: 2 in, 2 out]
          }
        }
        n764 = global read "Global.vi" "程序关闭"() -> (w74:bool)
      }
    }
  }
